vi "Main-GUI.vi"() -> ()   [LabVIEW 2021]
uses:
  Controls/Command_cluster.ctl
  Controls/Command_Enum.ctl
  Controls/AR-msg-variables.ctl
  Controls/AR-com-ports.ctl
  Controls/AR-instrument-refs.ctl
  C:/Projects/Automation/nLight Laser/nlight_dll/altaAPI.dll
  Automation/nLight Laser/nlight_dll/altaAPI.dll
  Controls/AR-axis-parameters.ctl
  Automation/Zaber Stage/Controls/Zaber-parameters.ctl
  Controls/AR-Interlock-Data.ctl
  Automation/nLight Laser/Controls/CW-Laser-params.ctl
  Automation/nLight Laser/Controls/Status-flags.ctl
  Automation/nLight Laser/Controls/nLight-beam-modes.ctl
  Controls/AR-Interlock-monitor-comands.ctl
  Automation/nLight Laser/Controls/nLight-wait-states.ctl
  <instrlib>/Zaber A Series/Zaber A Series.lvlib
panel:
  out "Accel Activ":bool
  out "msg-var at exit":T1={"Run Rcp"=FALSE, "Rcp Stopped"=FALSE, "Err Device"="", "Run Axis Loop"=TRUE}
  in  "Simulate Laser":bool
  out "error out":errorcluster
  in  "Axis params":T2={"X"={"Device (dev axis)"="1 3", "Lockstep Group (1)"=1, "Units"=enum."millimeters", "Microstep Size"=4.21875, "Move (units)"=1500.0, "Direction(-1,1)"=1, "Speed (units/s)"=0.0}, "Y"={"Device (dev axis)"="1", "Lockstep Group (1)"=1, "Units"=enum."millimeters", "Microstep Size"=0.496094, "Move (units)"=0.0, "Direction(-1,1)"=1, "Speed (units/s)"=0.0}}
  in  "Tab Control":T4(tab)=enum."SETTINGS (AXIS / SCRIPT)"
  in  "Start Y Position":dbl=85.0
  in  "Re-test gating":bool
  in  "X Axis Initial Test Parameters":T3={"Device (dev axis)"="1 3", "Lockstep Group (1)"=1, "Units"=enum."millimeters", "Microstep Size"=4.21875, "Move (units)"=1500.0, "Direction(-1,1)"=1, "Speed (units/s)"=0.0}
  out "MCU INLK":bool=TRUE
  in  "Init":bool=TRUE
  out "Laser OK":bool
  in  "Com ports":T5={"Zaber Com"="COM3", "MCU Com"="COM5", "Laser IP"="172.30.0.50", "Laser Com"=""}
  in  "Recipe (csv)":path=path "C:/Projects/Alpha Redux/test-scrypt-1.csv"
  out "Zaber OK":bool=TRUE
  out "Controll Interface":i32(ring) items=["HW", "API", "CLI", "INET, CONTROL_INT_MASK"]
  out "External Gate":bool
  out "Profile Mode":bool
  out "Gating Timedout":bool
  out "X Position Triggered":dbl
  out "Delta Time (mS)":dbl
  out "MCU Gating Flags":T6
  in  "Save script":bool
  in  "Load script":bool
  in  "Script":T7[](array[typedef])=[{"Step#"=10.0, "Commands"=enum."Home All", "Parameter1"=0.0, "Parameter2"=0.0, "Parameter3"=0.0}, {"Step#"=20.0, "Commands"=enum."Y Move Rel", "Parameter1"=20.0, "Parameter2"=1.0, "Parameter3"=0.0}, {"Step#"=30.0, "Commands"=enum."Wait", "Parameter1"=500.0, "Parameter2"=0.0, "Parameter3"=0.0}, {"Step#"=40.0, "Commands"=enum."X Move Abs", "Parameter1"=300.0, "Parameter2"=0.0, "Parameter3"=0.0}, {"Step#"=50.0, "Commands"=enum."Wait", "Parameter1"=1000.0, "Parameter2"=0.0, "Parameter3"=0.0}, {"Step#"=60.0, "Commands"=enum."Y Move Rel", "Parameter1"=10.0, "Parameter2"=-1.0, "Parameter3"=0.0}, {"Step#"=70.0, "Commands"=enum."Wait", "Parameter1"=500.0, "Parameter2"=0.0, "Parameter3"=0.0}, {"Step#"=80.0, "Commands"=enum."X Move Abs", "Parameter1"=50.0, "Parameter2"=0.0, "Parameter3"=0.0}, {"Step#"=90.0, "Commands"=enum."Wait", "Parameter1"=1000.0, "Parameter2"=0.0, "Parameter3"=0.0}, {"Step#"=100.0, "Commands"=enum."Repeat", "Parameter1"=20.0, "Parameter2"=5.0, "Parameter3"=0.0}, {"Step#"=110.0, "Commands"=enum."Y Move Abs", "Parameter1"=10.0, "Parameter2"=0.0, "Parameter3"=0.0}, {"Step#"=120.0, "Commands"=enum."End", "Parameter1"=0.0, "Parameter2"=0.0, "Parameter3"=0.0}]
  in  "Y Microstep Size":dbl=0.496094
  in  "X Microstep Size":dbl=4.21875
  in  "Y (dev axis)":string="1"
  in  "X (dev axis)":string="1 3"
  in  "Select Units":T9(ring)=enum."millimeters"
  in  "Zaber settings":bool
  out "Device Info":T10(array[cluster])=[{"Motion Type"="Linear", "Device Name"="X-MCC3 (rev 2) Controller + LRQ150BL-DE51T10A", "Microstep Size"=0.49609375000198436}, {"Motion Type"="Linear", "Device Name"="X-MCC3 (rev 2) Controller + LRQ150BL-DE51T10A", "Microstep Size"=0.49609375000198436}, {"Motion Type"="Linear", "Device Name"="X-MCC3 (rev 2) Controller + BLQ2095-E01T3A", "Microstep Size"=4.2187499996625}] {"Microstep Size" format="%#_6f"}
  out "Devices":string[](array[string])=["1"]
  out "Axis":string[](array[string])=["3"]
  out "Mode RDY":bool
  in  "Beam-profile(0-6)":T11
  in  "Speed mm/s":dbl=500.0
  in  "Clear":bool
  in  "Request":bool
  out "Gating Data":T12={"Application"="", "Msg#"=0, "uS time"=0, "Gate"=TRUE, "Head"=TRUE, "Head Old"=FALSE, "Chamber Ena"=FALSE, "Profiler Ena"=FALSE, "OPower Ena"=FALSE, "Gate Ena"=FALSE, "Time Delta (mS)"=0.0, "Head F Edge"=FALSE} {"Time Delta (mS)" format="%#_3f"}
  out "MCU Gating Raw Output":string
  out "Laser Msg Log":string
  in  "Laser Params":T13={"Power(W)"=30.0, "Duty(%)"=5.0, "Freq(Hz)"=1000.0}
  in  "SysON":bool
  in  "ENA":bool
  in  "Set Laser Params":bool caption="Set"
  out "Laser Status":T14
  out "Current Y Pos":dbl
  in  "Y Home":bool
  in  "Y Abs":bool
  in  "Y Abs Units":dbl=50.0
  out "Current X Pos":dbl=-3.9234375
  in  "Stop":bool
  in  "X Home":bool
  in  "X Abs":bool
  in  "X Abs Units":dbl=500.0
  in  "Y Units":dbl=1.0
  in  "X Units":dbl=10.0
  in  "Y Fw":bool
  in  "Y Back":bool
  in  "X Fw":bool
  in  "X Back":bool
  in  "EMIT!":bool
  in  "Head Flag\nLenght (mm)":dbl=100.0
  in  "Run script":bool
  in  "Stop":bool
  in  "Next":bool
  in  "Step":bool
  out "Y Position":dbl
  out "X Position":dbl
  out "Gate Trigger":cluster{dbl[], i16[]}(graph) caption="XY Graph - Light"
  out "Speeds (m/s)":dbl[](array[numeric])
  out "X Axis Pos/Speed":cluster{u32[], dbl[]}(graph) caption="XY Graph - Light"
  in  "Select":bool
  out "Laser Status":T14
  out "Laser Power (W)":dbl
  out "Laser Duty (%)":dbl
  out "Next command":T7
  in  "Target Time (s)":dbl=1.0
  in  "Accel COM":refnum<visa-resource-name>
  in  "Accel CSV File":path=path "C:/Users/cleanroom/Desktop/Accelerometer Files/Test1.csv"
  in  "Accel Ena":bool caption="ENABLE"
  out "File OK":bool
  out "Com\nError":bool
  out "Instr Refs":T15={"Zaber Com"="COM21", "MCU Com"="COM22", "LaserSysRef Out"=refnum, "LaserControl Ref Out"=refnum}
  in  "error in":errorcluster
  out "msg-var":T1={"Run Rcp"=FALSE, "Rcp Stopped"=FALSE, "Err Device"="", "Run Axis Loop"=TRUE}
  in  "Quit":bool
  out "Action":string="Quit"
  # "Emit not used\nwith EXT TRIG"
  # "EMIT! will work\nonly in GUI/CLI mode without EX GATE"
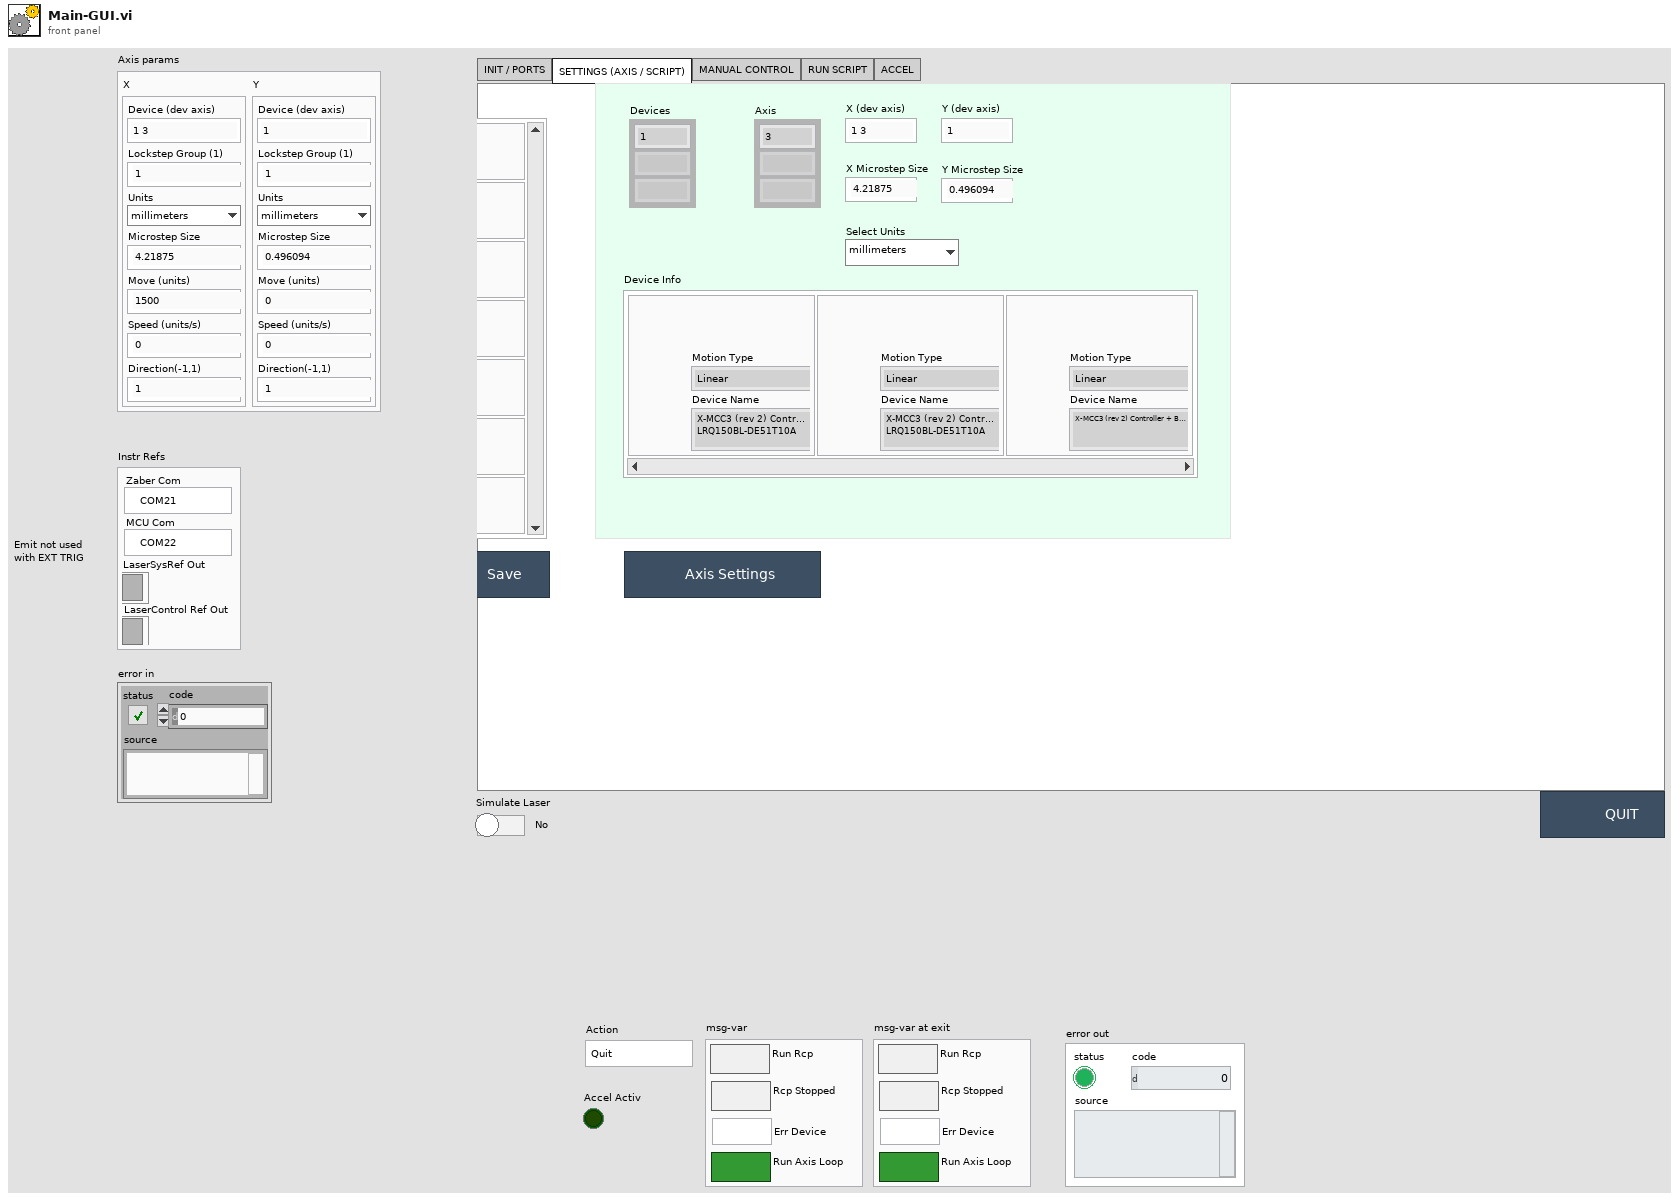
[diagram p1: front panel]
types:
  T1 = typedef "AR-msg-variables.ctl" = cluster{"Run Rcp":bool, "Rcp Stopped":bool, "Err Device":string, "Run Axis Loop":bool}
  T2 = typedef "AR-axis-parameters.ctl" = cluster{"X":T3, "Y":T3}
  T3 = typedef "Zaber-parameters.ctl" = cluster{"Device (dev axis)":string, "Lockstep Group (1)":u8, "Units":enum16{"microsteps", "microns", "millimeters", "inches", "degrees"}, "Microstep Size":dbl, "Move (units)":dbl, "Direction(-1,1)":i32, "Speed (units/s)":dbl}
  T4 = enum32{"INIT / PORTS", "SETTINGS (AXIS / SCRIPT)", "MANUAL CONTROL", "RUN SCRIPT", "ACCEL"}
  T5 = typedef "AR-com-ports.ctl" = cluster{"Zaber Com":refnum<visa-resource-name>, "MCU Com":refnum<visa-resource-name>, "Laser IP":string, "Laser Com":refnum<visa-resource-name>}
  T6 = cluster{"Chamber Ena":bool, "Profiler Ena":bool, "OPower Ena":bool}
  T7 = typedef "Command_cluster.ctl" = cluster{"Step#":dbl, "Commands":T8, "Parameter1":dbl, "Parameter2":dbl, "Parameter3":dbl}
  T8 = typedef "Command_Enum.ctl" = enum16{"End", "Home All", "X Home", "Y Home", "X Move Rel", "X Move Abs", "Y Move Rel", "Y Move Abs", "Wait", "Repeat", "Reset Intlk Timer", "Laser Sys ON", "Laser ENA"}
  T9 = enum16{"microsteps", "microns", "millimeters", "inches", "degrees"}
  T10 = cluster{"Motion Type":string, "Device Name":string, "Microstep Size":dbl}[]
  T11 = typedef "nLight-beam-modes.ctl" = enum32{"0/100 single-mode", "30/70", "40/60", "50/50", "60/40", "80/20", "90/10 max donut"}
  T12 = typedef "AR-Interlock-Data.ctl" = cluster{"Application":string, "Msg#":i32, "uS time":u32, "Gate":bool, "Head":bool, "Head Old":bool, "Chamber Ena":bool, "Profiler Ena":bool, "OPower Ena":bool, "Gate Ena":bool, "Time Delta (mS)":dbl, "Head F Edge":bool}
  T13 = typedef "CW-Laser-params.ctl" = cluster{"Power(W)":dbl, "Duty(%)":dbl, "Freq(Hz)":dbl}
  T14 = typedef "Status-flags.ctl" = cluster{"SystemOn":bool, "Enabled":bool, "LaserOn":bool, "Standby":bool, "Interlock":bool, "Error":bool, "Warning":bool, "Fault":bool}
  T15 = typedef "AR-instrument-refs.ctl" = cluster{"Zaber Com":refnum<visa-resource-name>, "MCU Com":refnum<visa-resource-name>, "LaserSysRef Out":refnum<k24>, "LaserControl Ref Out":refnum<k24>}
  T16 = enum32{"INIT / PORTS", "SETTINGS (AXIS / SCRIPT)", "MANUAL CONTROL", "RUN SCRIPT"}
  T17 = enum32{"Page Enabled", "Page Disabled", "Page Disabled & Grayed"}
  T18 = typedef "AR-Interlock-monitor-comands.ctl" = enum16{"Init", "Request", "Poll Serial", "Close", "Clear Data"}
  T19 = enum8{"Enabled", "Disabled", "Disabled and Grayed Out"}
  T20 = typedef "nLight-wait-states.ctl" = enum16{"Wait SysON", "Wait ENA", "Wait SysOFF", "Wait DIS", "No Wait"}
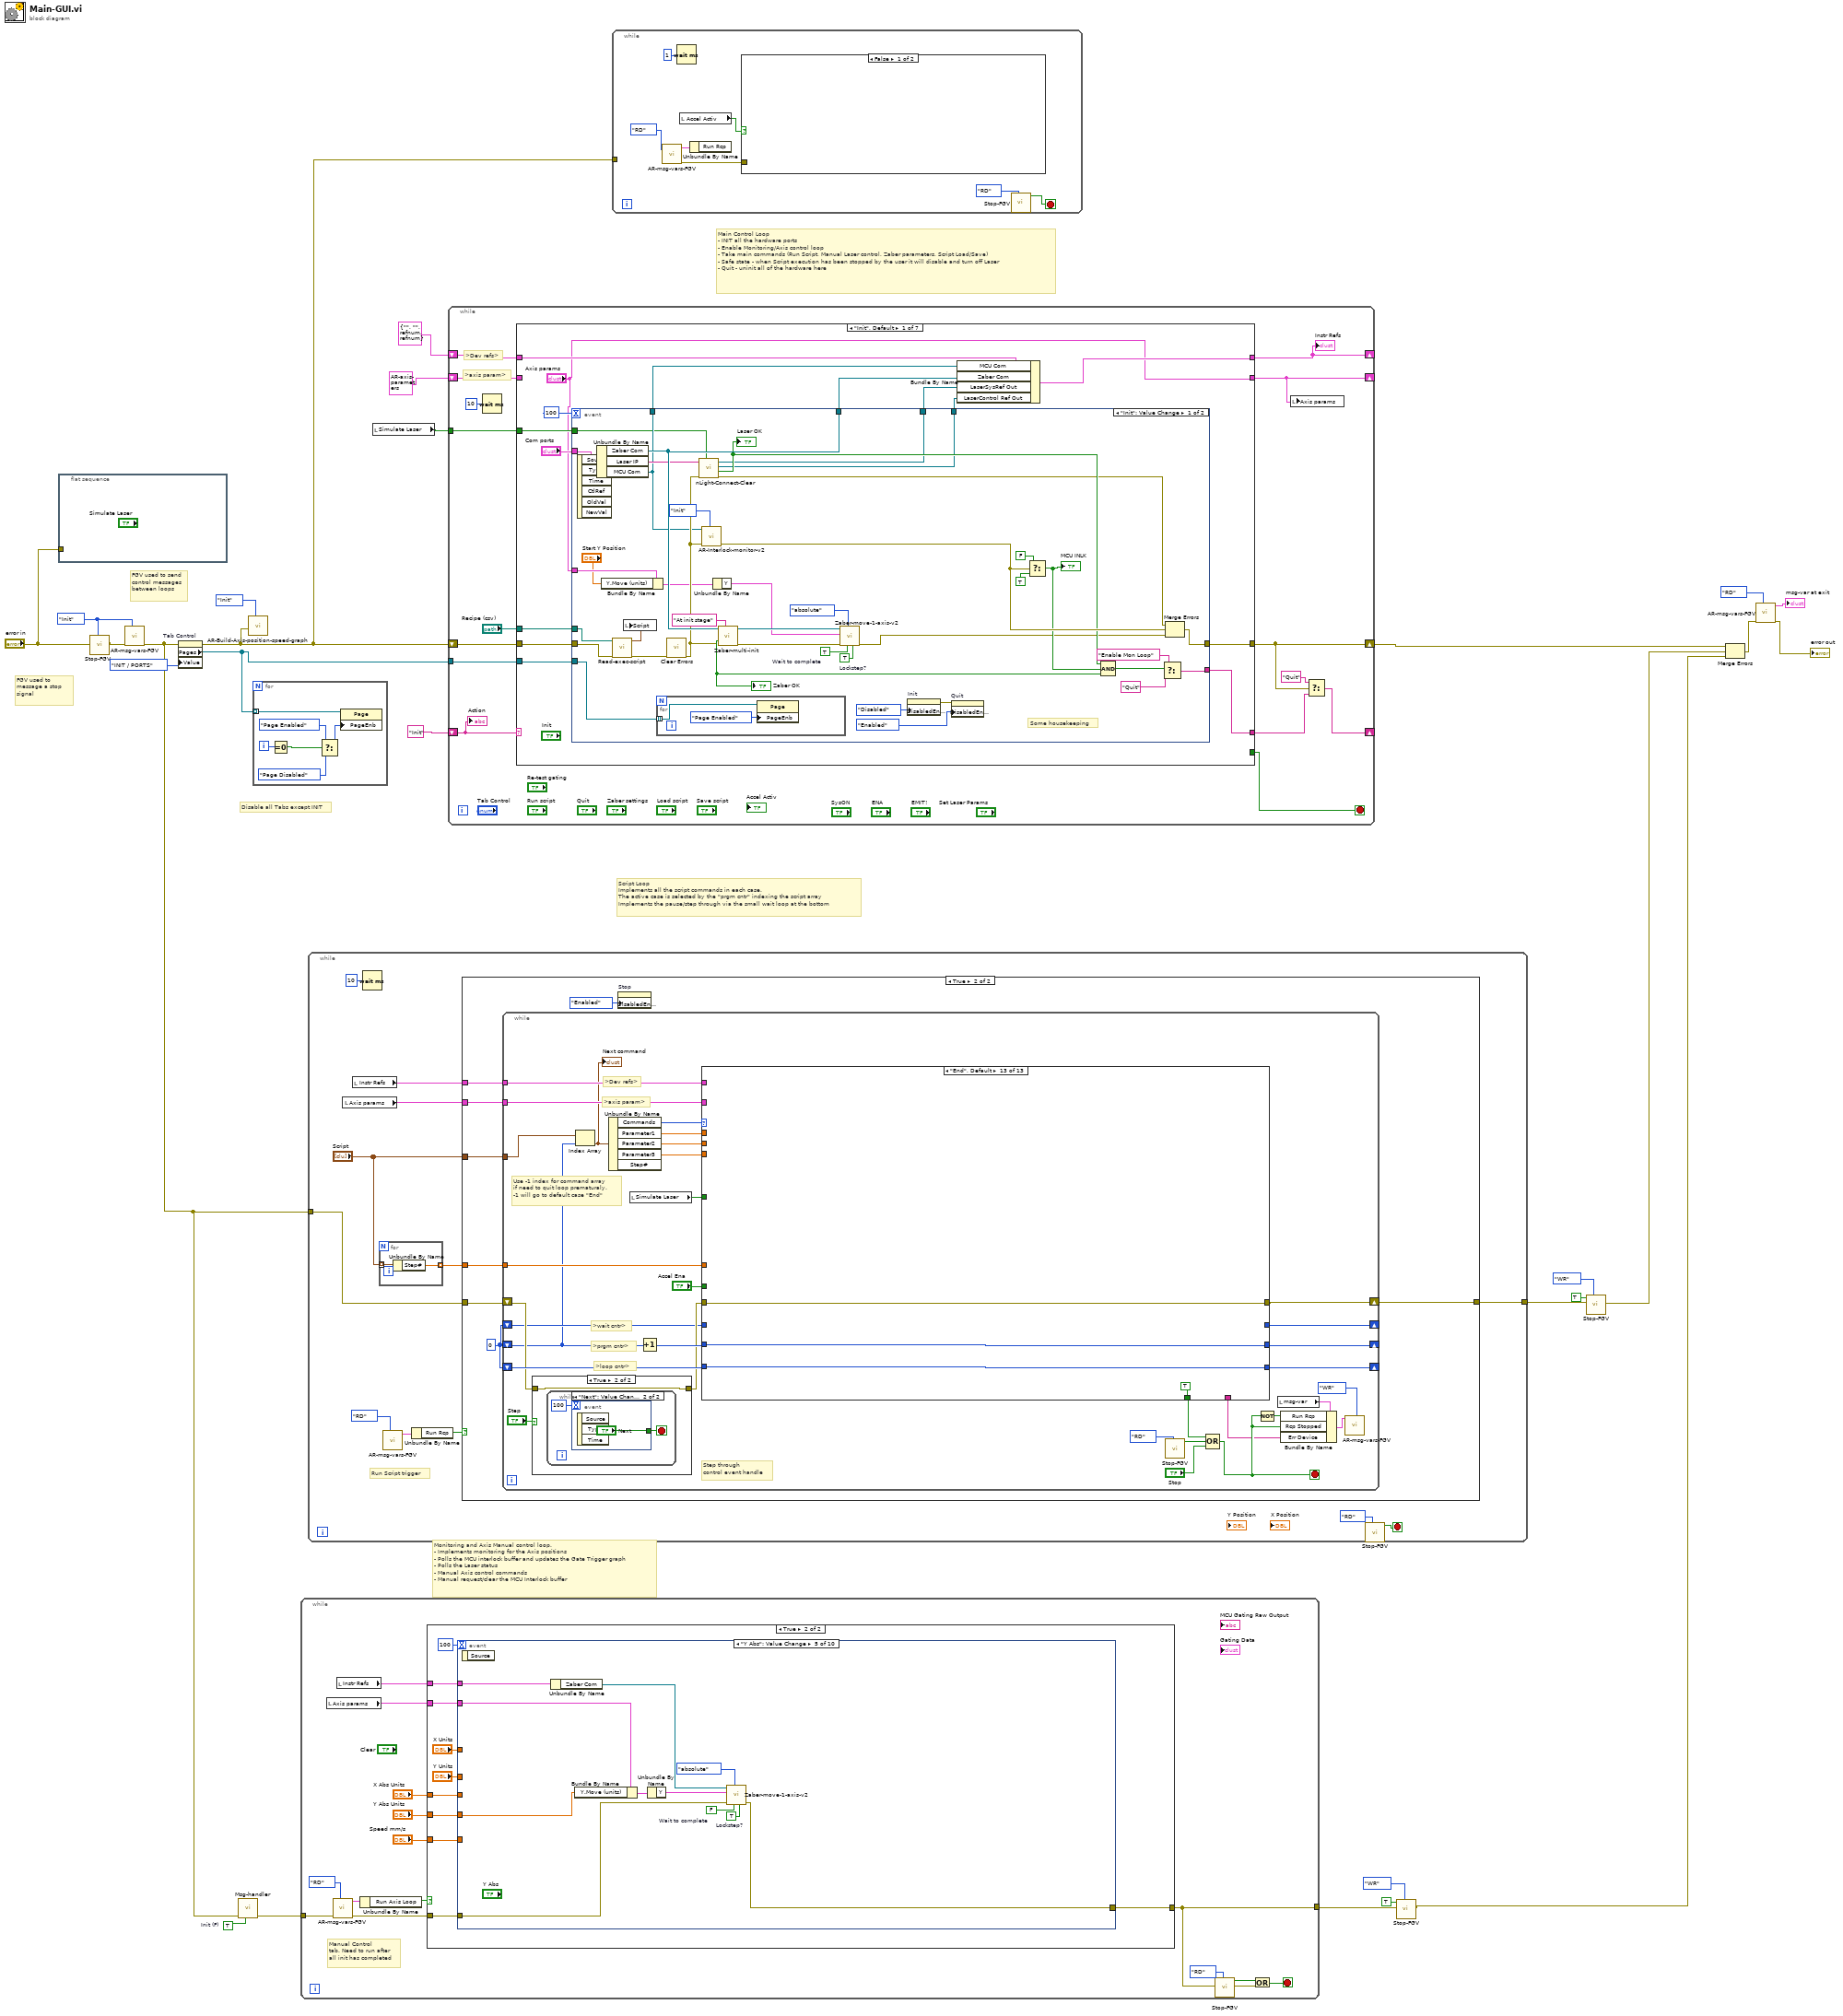
[diagram p0: block diagram]
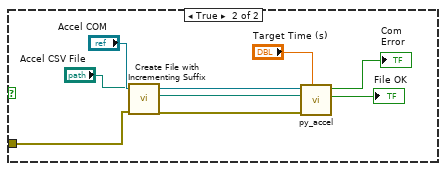
[diagram p2: hidden frame]
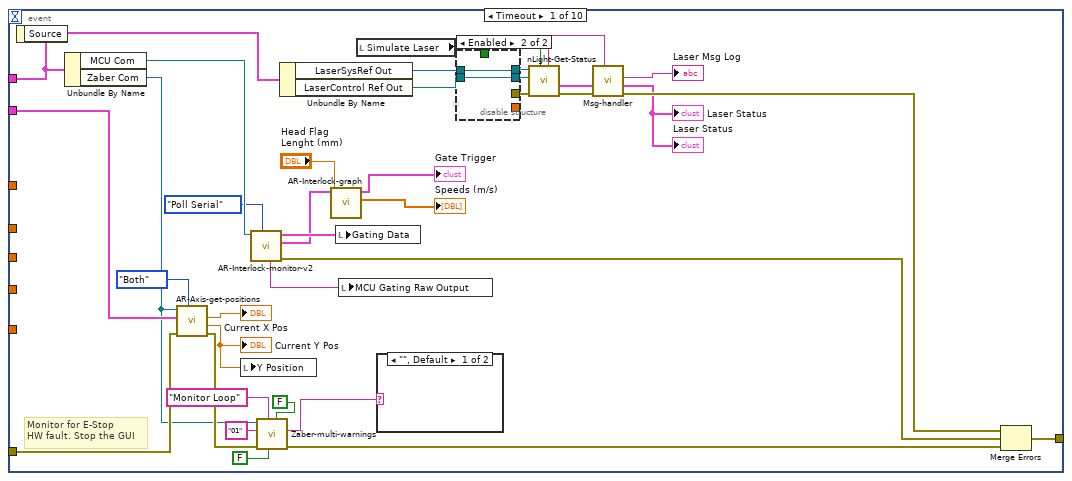
[diagram p4: hidden frame]
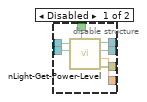
[diagram p5: hidden frame]
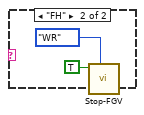
[diagram p6: hidden frame]
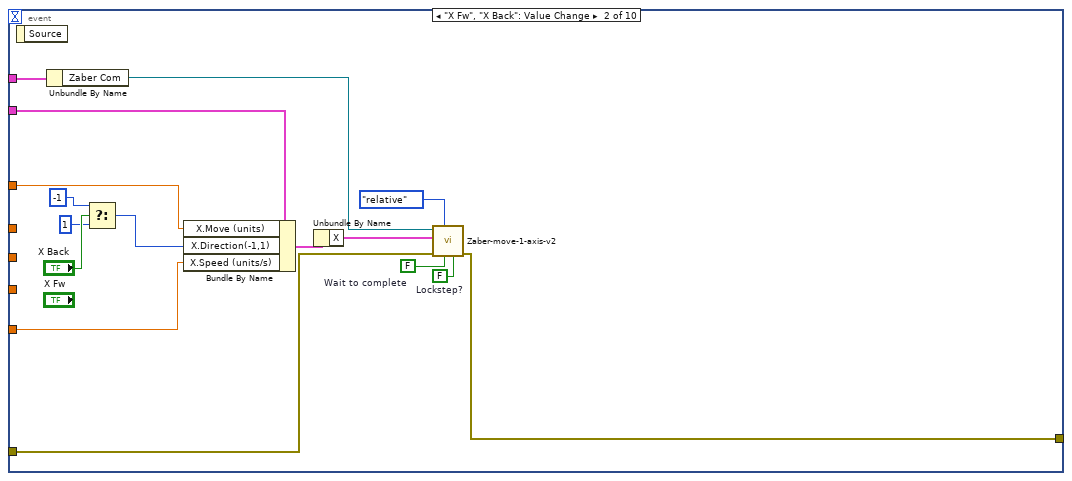
[diagram p7: hidden frame]
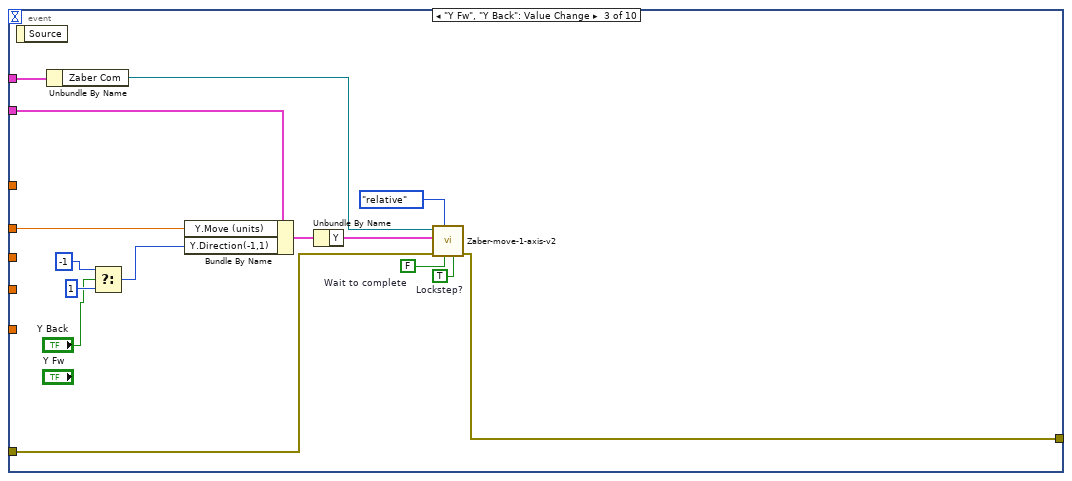
[diagram p8: hidden frame]
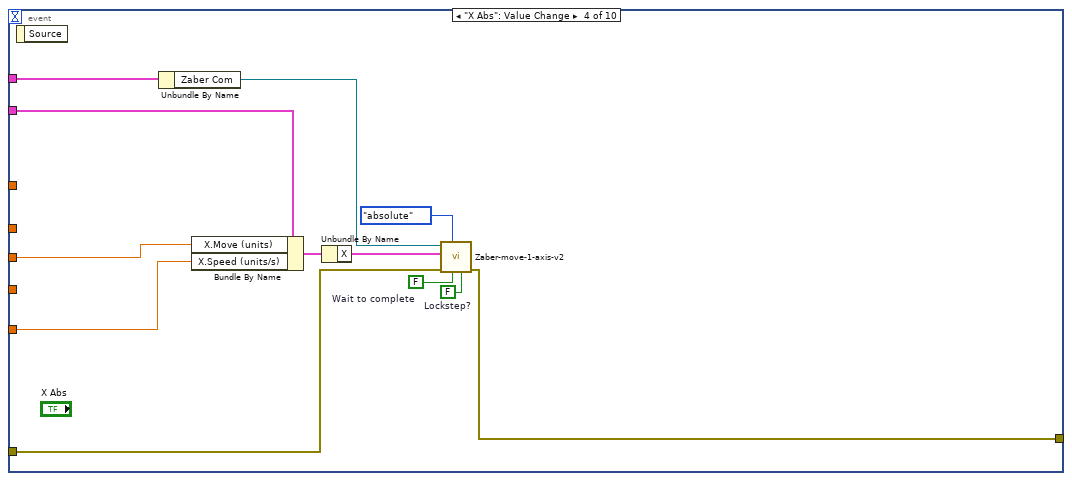
[diagram p9: hidden frame]
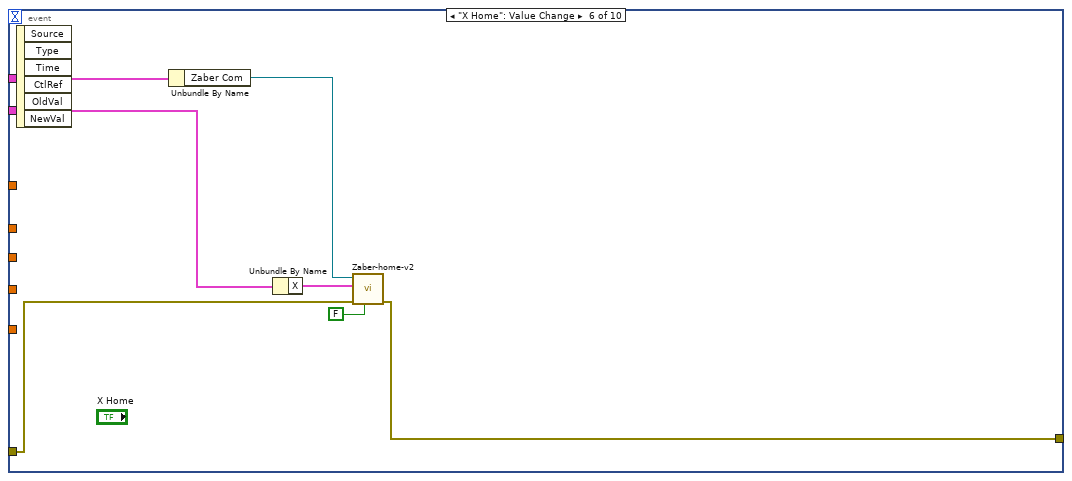
[diagram p10: hidden frame]
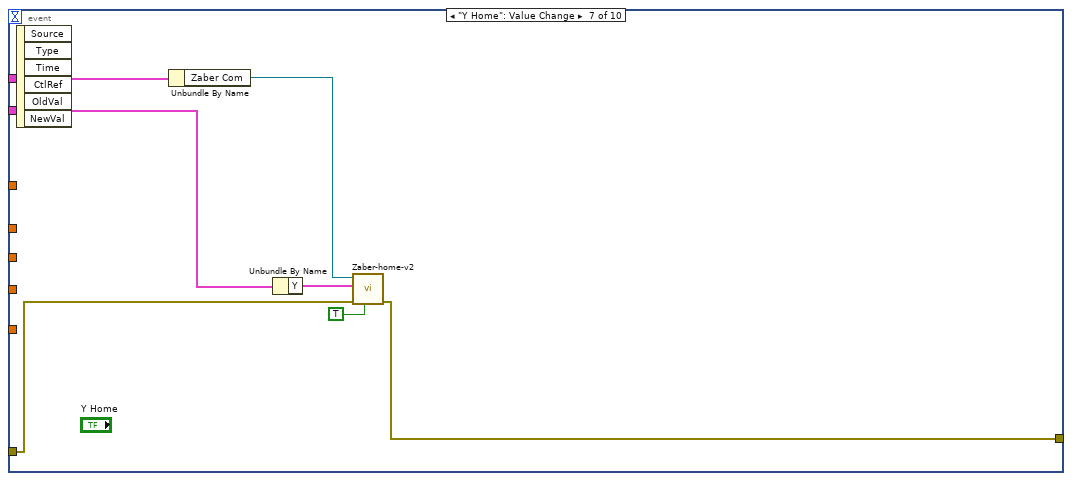
[diagram p11: hidden frame]
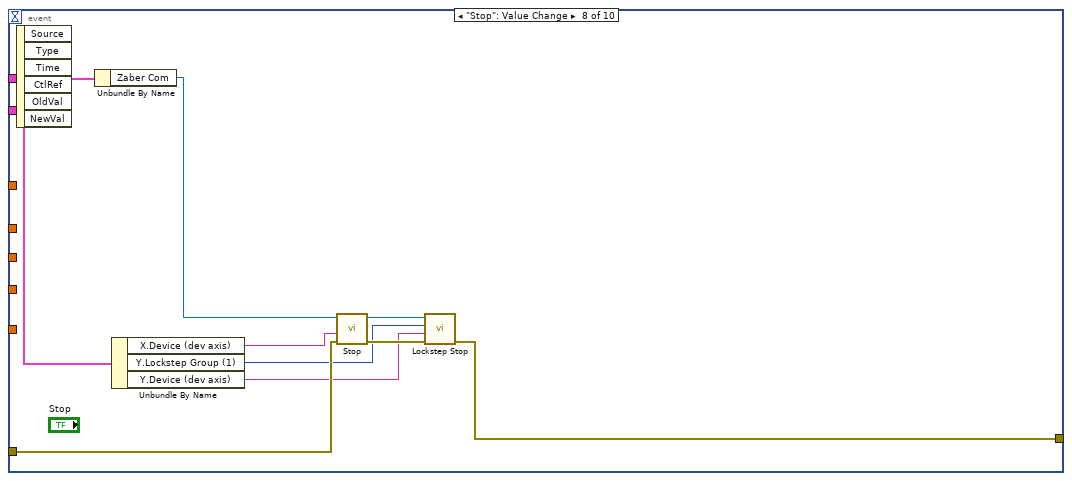
[diagram p12: hidden frame]
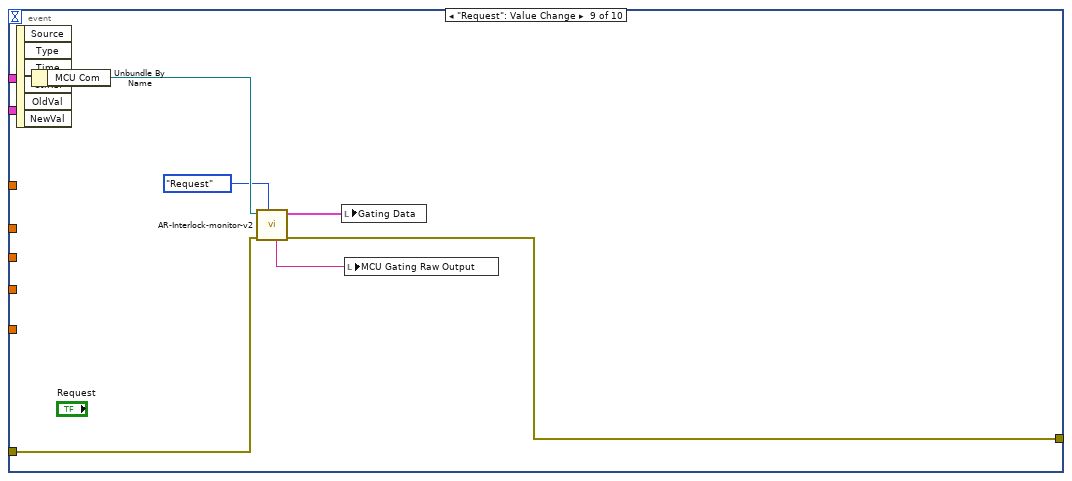
[diagram p13: hidden frame]
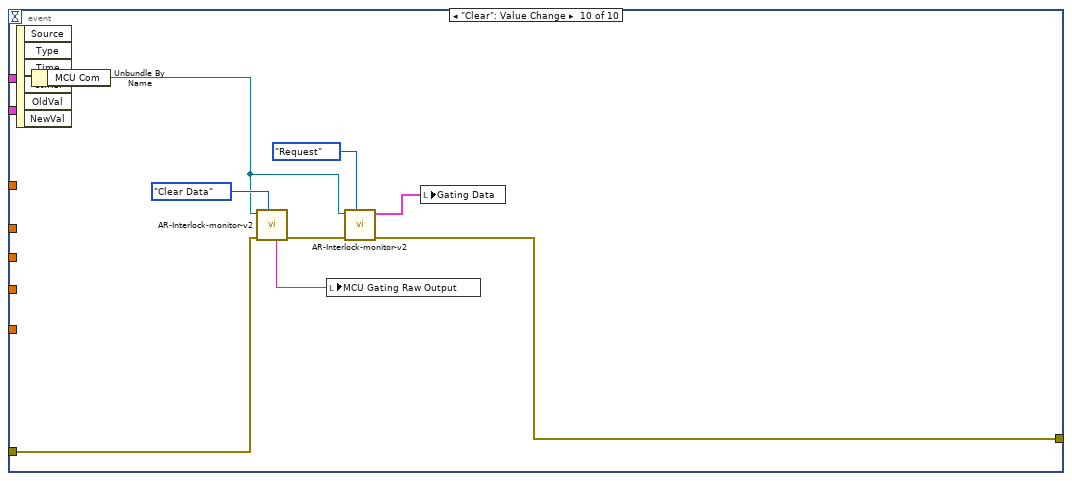
[diagram p14: hidden frame]
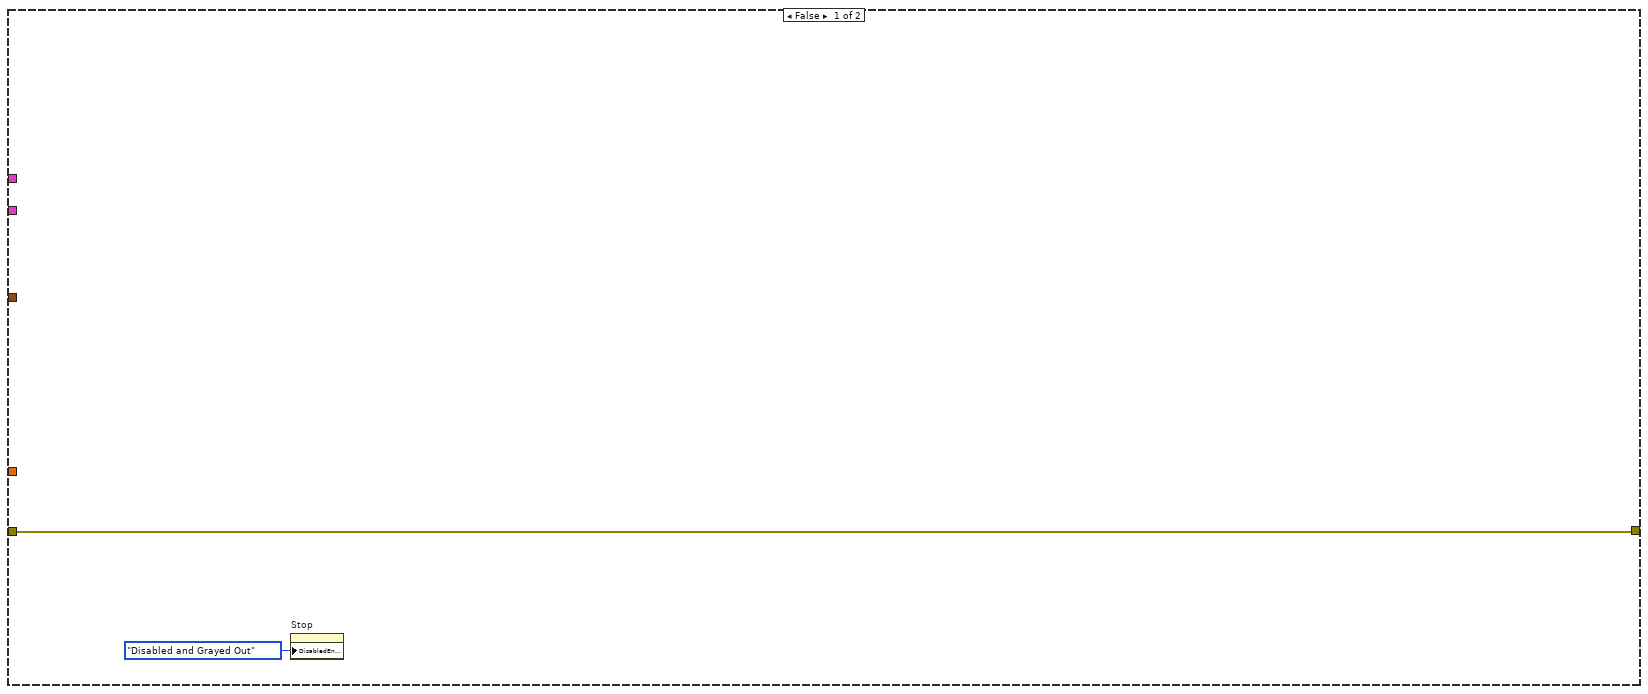
[diagram p15: hidden frame]
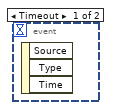
[diagram p17: hidden frame]
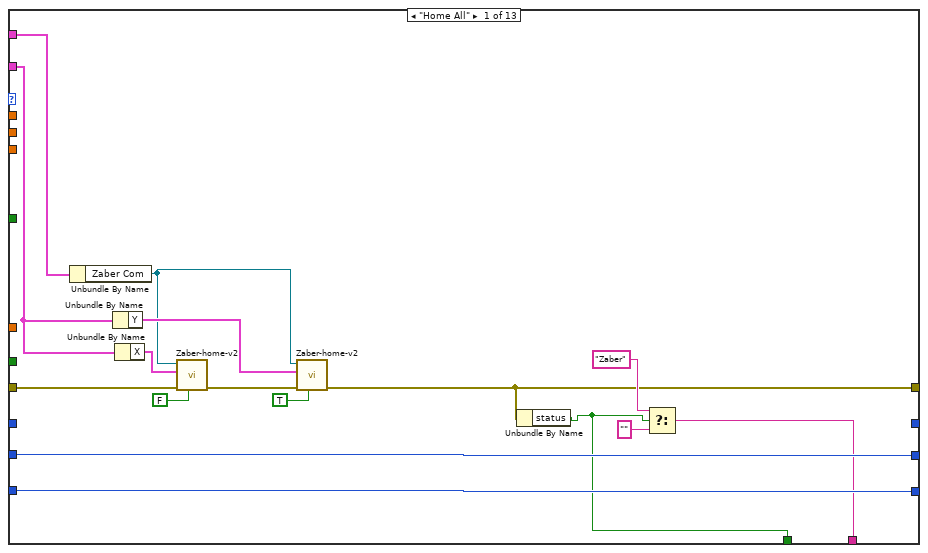
[diagram p18: hidden frame]
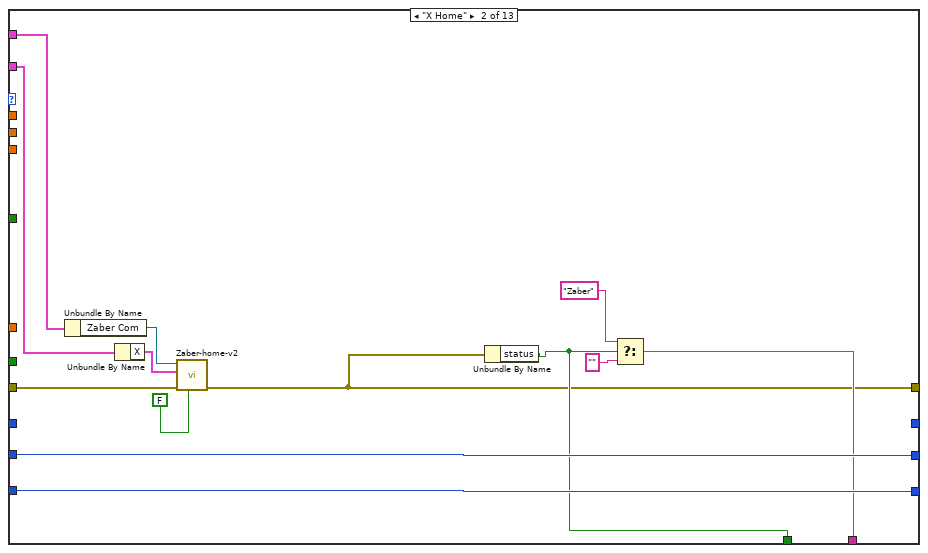
[diagram p19: hidden frame]
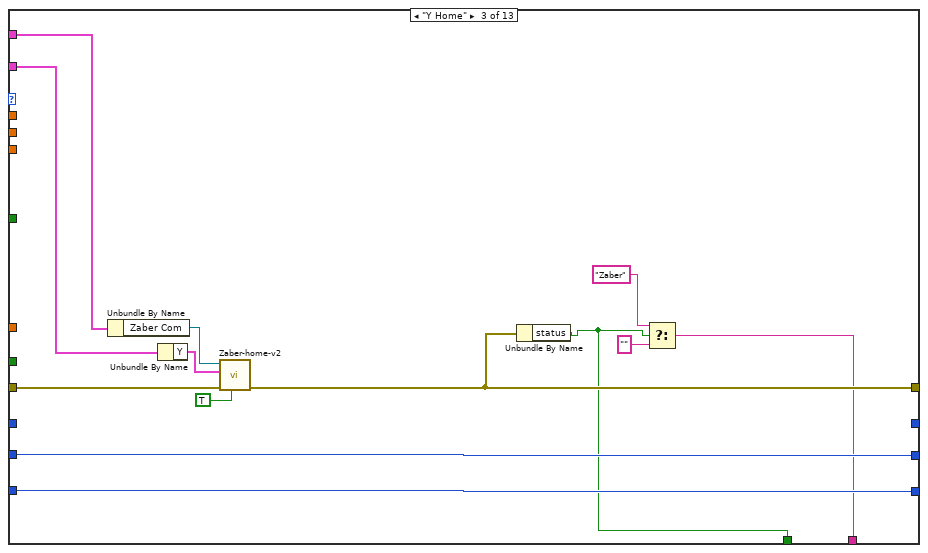
[diagram p20: hidden frame]
diagram:
  w19 = TRUE  # Init (F)
  w25 = enum16{"Init", "WR", "RD"}."Init" ("Action (RD)")
  # "Monitoring and Axis Manual control loop.\n- Implements monitoring for the Axis positions\n- Polls the MCU interlock buffer and updates the Gate Trigger graph\n- Polls the Laser status\n- Manual Axis control commands\n- Manual request/clear the MCU Interlock buffer"
  # "Main Control Loop\n- INIT all the hardware ports \n- Enable Monitoring/Axis control loop\n- Take main commands (Run Script, Manual Laser control, Zaber parameters, Script Load/Save)\n- Safe state - when Script execution has been stopped by the user it will disable and turn off Laser\n- Quit - uninit all of the hardware here"
  # "Disable all Tabs except INIT"
  # "FGV used to send control messages between loops"
  # "FGV used to \nmessage a stop\nsignal"
  # "Script Loop\nImplements all the script commands in each case.\nThe active case is selected by the \"prgm cntr\" indexing the script array\nImplements the pause/step through via the small wait loop at the bottom"
  n1 = flat-sequence {
    tunnel: "error in" -> [_]
    frame #0 {
    }
  }
  n2 = call "Stop-FGV.vi"("Action (RD)"=w25, "error in"="error in") -> ("error out"=w26:errorcluster)  [unwired: 8 in, 1 out]
  n3 = call "AR-msg-vars-FGV.vi"("Action"=w25, "error in"=w26) -> ("error out"=w18:errorcluster)  [unwired: 8 in, 1 out]
  n4 = property on="Tab Control" class="TabCtl (strict)"(error in=w18, "Value"=T16."INIT / PORTS" ("Tab Control")) -> (error out=w1:errorcluster, "Pages"=w22:refnum<vi>[])  [unwired: 1 in, 1 out]
  n5 = call "Msg-handler.vi"("Init (F)"=w19, "error in"=w18) -> ("error out"=w17:errorcluster)  [unwired: 6 in, 3 out]
  n6 = call "AR-Build-Axis-position-speed-graph.vi"("Action"=enum16{"Init", "WR", "RD"}."Init", "error in (no error)"=w1) -> ()  [unwired: 9 in, 1 out]
  n7 = for {
    tunnel: w22 -> [w33] mode=indexing
    i -> [w32]
    n8 = Equal To 0?(x=w32) -> (x = 0?=w31:bool)
    n9 = Select(t=T17."Page Enabled" ("Page Enabled State"), s=w31, f=T17."Page Disabled" ("Page Enabled State")) -> (s? t:f=w28:T17)
    n10 = property class="Page"(reference=w33, "PageEnb"=w28) -> ()  [unwired: 1 in, 2 out]
  }
  n11 = while {
    tunnel: w17 -> [w42]
    tunnel: [w36] -> w11
    stop <- w40 stop-if-true
    # "Manual Control\ntab. Need to run after\nall init has completed"
    n12 = local read "Axis params"() -> (w43:T2)
    n13 = call "AR-msg-vars-FGV.vi"("Action"=enum16{"Init", "WR", "RD"}."RD", "error in"=w42) -> ("error out"=w41:errorcluster, "msg-var"=w47:T1)  [unwired: 8 in]
    n14 = local read "Instr Refs"() -> (w44:T15)
    n15 = Unbundle By Name(w47) -> ("Run Axis Loop"=w45:bool)
    n16 = case shown="True" w45 {
      tunnel: w44 -> [_ w59]
      tunnel: w43 -> [_ w58]
      tunnel: w41 -> [w49 w57]
      tunnel: [w49 w56] -> w36
      tunnel: "X Abs Units" -> [_ w52]
      tunnel: "Y Abs Units" -> [_ w51]
      tunnel: "Speed mm/s" -> [_ w50]
      frame False {
      }
      frame True {
        # "Run Sequence"
        n17 = event shown="[4] \"Y Abs\": Value Change" {
          selector: _ -> [_ _ _ _ _ _ _ _ _ _]
          dyn-events: _ -> [_ _ _ _ _ _ _ _ _ _]
          timeout: 100 -> [_ _ _ _ _ _ _ _ _ _]
          tunnel: w59 -> [w78 w112 w128 w143 w154 w164 w171 w184 w187 w199]
          tunnel: w58 -> [w94 w113 w129 w144 w155 w163 w170 w178 _ _]
          tunnel: w57 -> [w93 w110 w126 w140 w152 w162 w169 w181 w189 w200]
          tunnel: [w88 w109 w125 w139 w151 w161 w168 w179 w188 w196] -> w56
          tunnel: "Y Units" -> [_ _ w123 _ _ _ _ _ _ _]
          tunnel: "X Units" -> [_ w108 _ _ _ _ _ _ _ _]
          tunnel: w52 -> [_ _ _ w141 _ _ _ _ _ _]
          tunnel: w51 -> [_ _ _ _ w150 _ _ _ _ _]
          tunnel: w50 -> [_ w107 _ w138 _ _ _ _ _ _]
          event Timeout {
            # "Monitor for E-Stop\nHW fault. Stop the GUI"
            n18 = event-data() -> ()  [unwired: 1 in, 1 out]
            n19 = Unbundle By Name(w78) -> ("MCU Com"=w91:refnum<visa-resource-name>, "Zaber Com"=w66:refnum<visa-resource-name>)
            n20 = call "AR-Axis-get-positions.vi"("Select"=enum16{"X Axis", "Y Axis", "Both"}."Both", "error in"=w93, "Axis params"=w94, "Port In"=w66) -> ("error out"=w67:errorcluster, "Y Pos"=w82:dbl, "X Pos"=→"Current X Pos":dbl)  [unwired: 4 in, 1 out]
            "Current Y Pos" <- w82
            n21 = local write "Y Position"(w82) -> ()
            n22 = call "AR-Interlock-monitor-v2.vi"("Action"=AR-Interlock-monitor-comands."Poll Serial", "Inlk Com"=w91) -> ("error out"=w89:errorcluster, "Intlk Data Array"=w85:T12[], "Intlk Data"=w86:T12, "Raw Output"=w87:string)  [unwired: 5 in, 1 out]
            n23 = call "Zaber-multi-warnings.vi"("Log?"=FALSE, "Msg?"=FALSE, "LogSource"="Monitor Loop", "error in"=w67, "Device"="01", "Com Port"=w66) -> ("error out"=w62:errorcluster, "Warning Flag"=w61:string)  [unwired: 2 in, 2 out]
            n24 = Unbundle By Name(w78) -> ("LaserSysRef Out"=w74:refnum<k24>, "LaserControl Ref Out"=w72:refnum<k24>)
            n25 = call "AR-Interlock-graph.vi"("Flag Lenght (mm)"="Head Flag\nLenght (mm)", "Intlk Data Array"=w85) -> ("Speeds (m/s)"=→"Speeds (m/s)":dbl[], "Gate"=→"Gate Trigger":cluster{dbl[], i16[]})  [unwired: 7 in, 1 out]
            n26 = local write "Gating Data"(w86) -> ()
            n27 = local write "MCU Gating Raw Output"(w87) -> ()
            n28 = local read "Simulate Laser"() -> (w69:bool)
            n29 = case shown="\"\", Default" w61 {
              frame "", Default {
              }
              frame "FH" {
                n30 = call "Stop-FGV.vi"("Action (RD)"=enum16{"Init", "WR", "RD"}."WR", "Action"=TRUE) -> ()  [unwired: 8 in, 2 out]
              }
            }
            n31 = disable-structure shown="Enabled" {
              disable-tunnel: w74 -> [w102 w103]
              disable-tunnel: [w101 w103] -> w73
              disable-tunnel: w72 -> [w100 w104]
              disable-tunnel: [w99 w104] -> w71
              disable-tunnel: [w98 _] -> w70
              disable-tunnel: [w97 _] -> _
              disable-tunnel: w69 -> [w96 _]
              frame Disabled {
                n32 = call "nLight-Get-Power-Level.vi"("Simulate (F)"=w96, "LaserControl Ref"=w100, "LaserSysRef"=w102) -> ("error out"=w98:errorcluster, "PowerOutput"=w97:dbl, "LaserControl Ref Out"=w99:refnum<k24>, "LaserSysRef Out"=w101:refnum<k24>)  [unwired: 5 in]
              }
              frame Enabled {
              }
            }
            n33 = call "nLight-Get-Status.vi"("Simulate (F)"=w69, "error in"=w70, "LaserControl Ref"=w71, "LaserSysRef"=w73) -> ("error out"=w79:errorcluster, "Status-flags"=w80:T14, "Msg"=w81:string)  [unwired: 2 in, 3 out]
            n34 = call "Msg-handler.vi"("Msg"=w81, "error in"=w79, "Status-flags"=w80) -> ("error out"=w76:errorcluster, "Status-flags Out"=→"Laser Status" →"Laser Status":T14, "Msg log"=→"Laser Msg Log":string)  [unwired: 5 in, 1 out]
            n35 = Merge Errors(w76, w89, w62) -> (w88:errorcluster)
          }
          event "X Fw", "X Back": Value Change {
            w117 = FALSE  # Wait to complete
            w118 = FALSE  # Lockstep?
            n36 = event-data() -> ()  [unwired: 1 in, 1 out]
            n37 = Unbundle By Name(w112) -> ("Zaber Com"=w111:refnum<visa-resource-name>)
            n38 = Select(t=-1 ("Direction(-1,1)"), s="X Back", f=1) -> (s? t:f=w121:i32)
            n39 = Bundle By Name(cluster=w113, "X.Move (units)"=w108, "X.Direction(-1,1)"=w121, "X.Speed (units/s)"=w107) -> (w114:T2)
            n40 = Unbundle By Name(w114) -> ("X"=w115:T3)
            n41 = call "Zaber-move-1-axis-v2.vi"("Lockstep?"=w118, "Wait to complete"=w117, "Movement Type"=enum16{"relative", "absolute"}."relative", "error in"=w110, "Zaber parameters"=w115, "Port In"=w111) -> ("error out"=w109:errorcluster)  [unwired: 3 in, 2 out]
          }
          event "Y Fw", "Y Back": Value Change {
            w133 = FALSE  # Wait to complete
            w134 = TRUE  # Lockstep?
            n42 = event-data() -> ()  [unwired: 1 in, 1 out]
            n43 = Unbundle By Name(w128) -> ("Zaber Com"=w127:refnum<visa-resource-name>)
            n44 = Select(t=-1 ("Direction(-1,1)"), s="Y Back", f=1) -> (s? t:f=w137:i32)
            n45 = Bundle By Name(cluster=w129, "Y.Move (units)"=w123, "Y.Direction(-1,1)"=w137) -> (w130:T2)
            n46 = Unbundle By Name(w130) -> ("Y"=w131:T3)
            n47 = call "Zaber-move-1-axis-v2.vi"("Lockstep?"=w134, "Wait to complete"=w133, "Movement Type"=enum16{"relative", "absolute"}."relative", "error in"=w126, "Zaber parameters"=w131, "Port In"=w127) -> ("error out"=w125:errorcluster)  [unwired: 3 in, 2 out]
          }
          event "X Abs": Value Change {
            w148 = FALSE  # Wait to complete
            w149 = FALSE  # Lockstep?
            n48 = event-data() -> ()  [unwired: 1 in, 1 out]
            n49 = Unbundle By Name(w143) -> ("Zaber Com"=w142:refnum<visa-resource-name>)
            n50 = Bundle By Name(cluster=w144, "X.Move (units)"=w141, "X.Speed (units/s)"=w138) -> (w145:T2)
            n51 = Unbundle By Name(w145) -> ("X"=w146:T3)
            n52 = call "Zaber-move-1-axis-v2.vi"("Lockstep?"=w149, "Wait to complete"=w148, "Movement Type"=enum16{"relative", "absolute"}."absolute", "error in"=w140, "Zaber parameters"=w146, "Port In"=w142) -> ("error out"=w139:errorcluster)  [unwired: 3 in, 2 out]
          }
          event "Y Abs": Value Change {
            w159 = FALSE  # Wait to complete
            w160 = TRUE  # Lockstep?
            n53 = event-data() -> ()  [unwired: 1 in, 1 out]
            n54 = Unbundle By Name(w154) -> ("Zaber Com"=w153:refnum<visa-resource-name>)
            n55 = Bundle By Name(cluster=w155, "Y.Move (units)"=w150) -> (w156:T2)
            n56 = Unbundle By Name(w156) -> ("Y"=w157:T3)
            n57 = call "Zaber-move-1-axis-v2.vi"("Lockstep?"=w160, "Wait to complete"=w159, "Movement Type"=enum16{"relative", "absolute"}."absolute", "error in"=w152, "Zaber parameters"=w157, "Port In"=w153) -> ("error out"=w151:errorcluster)  [unwired: 3 in, 2 out]
          }
          event "X Home": Value Change {
            n58 = event-data() -> ()  [unwired: 1 in, 6 out]
            n59 = Unbundle By Name(w164) -> ("Zaber Com"=w165:refnum<visa-resource-name>)
            n60 = Unbundle By Name(w163) -> ("X"=w166:T3)
            n61 = call "Zaber-home-v2.vi"("Lockstep?"=FALSE, "error in"=w162, "Zaber parameters"=w166, "Com Port"=w165) -> ("error out"=w161:errorcluster)  [unwired: 5 in, 2 out]
          }
          event "Y Home": Value Change {
            n62 = event-data() -> ()  [unwired: 1 in, 6 out]
            n63 = Unbundle By Name(w171) -> ("Zaber Com"=w172:refnum<visa-resource-name>)
            n64 = Unbundle By Name(w170) -> ("Y"=w173:T3)
            n65 = call "Zaber-home-v2.vi"("Lockstep?"=TRUE, "error in"=w169, "Zaber parameters"=w173, "Com Port"=w172) -> ("error out"=w168:errorcluster)  [unwired: 5 in, 2 out]
          }
          event "Stop": Value Change {
            n66 = event-data() -> ()  [unwired: 1 in, 6 out]
            n67 = Unbundle By Name(w184) -> ("Zaber Com"=w183:refnum<visa-resource-name>)
            n68 = Unbundle By Name(w178) -> ("X.Device (dev axis)"=w177:string, "Y.Lockstep Group (1)"=w176:u8, "Y.Device (dev axis)"=w175:string)
            n69 = call <instrlib>:"Stop.vi"("error in (no error)"=w181, "Device and Axis"=w177, "VISA resource name"=w183) -> ("error out"=w180:errorcluster, "VISA resource name out"=w182:refnum<visa-resource-name>)  [unwired: 7 in]
            n70 = call <instrlib>:"Lockstep Stop.vi"("error in (no error)"=w180, "Device Number"=w175, "Lockstep Group (1)"=w176, "VISA resource name"=w182) -> ("error out"=w179:errorcluster)  [unwired: 6 in, 1 out]
          }
          event "Request": Value Change {
            n71 = event-data() -> ()  [unwired: 1 in, 6 out]
            n72 = Unbundle By Name(w187) -> ("MCU Com"=w186:refnum<visa-resource-name>)
            n73 = call "AR-Interlock-monitor-v2.vi"("Action"=AR-Interlock-monitor-comands."Request", "error in"=w189, "Inlk Com"=w186) -> ("error out"=w188:errorcluster, "Intlk Data"=w190:T12, "Raw Output"=w191:string)  [unwired: 4 in, 2 out]
            n74 = local write "Gating Data"(w190) -> ()
            n75 = local write "MCU Gating Raw Output"(w191) -> ()
          }
          event "Clear": Value Change {
            n76 = event-data() -> ()  [unwired: 1 in, 6 out]
            n77 = Unbundle By Name(w199) -> ("MCU Com"=w195:refnum<visa-resource-name>)
            n78 = call "AR-Interlock-monitor-v2.vi"("Action"=AR-Interlock-monitor-comands."Clear Data" ("t"), "error in"=w200, "Inlk Com"=w195) -> ("error out"=w197:errorcluster, "Raw Output"=w192:string)  [unwired: 4 in, 3 out]
            n79 = local write "MCU Gating Raw Output"(w192) -> ()
            n80 = call "AR-Interlock-monitor-v2.vi"("Action"=AR-Interlock-monitor-comands."Request", "error in"=w197, "Inlk Com"=w195) -> ("error out"=w196:errorcluster, "Intlk Data"=w193:T12)  [unwired: 4 in, 3 out]
            n81 = local write "Gating Data"(w193) -> ()
          }
        }
      }
    }
    n82 = call "Stop-FGV.vi"("Action (RD)"=enum16{"Init", "WR", "RD"}."RD", "error in"=w36) -> ("error out"=w34:errorcluster, "Out"=w35:bool)  [unwired: 8 in]
    n83 = Or(x=w35, y=w34) -> (x .or. y?=w40:bool)
  }
  n84 = while {
    tunnel: w18 -> [w209]
    tunnel: [w201] -> w16
    stop <- w212 stop-if-true
    # "Run Script trigger"
    n85 = local read "Axis params"() -> (w205:T2)
    n86 = local read "Instr Refs"() -> (w206:T15)
    n87 = Wait (ms)(milliseconds to wait=u32 10) -> ()  [unwired: 1 out]
    n88 = for {
      tunnel: "Script" -> [w515] mode=indexing
      tunnel: [w514] -> w204 mode=indexing
      n89 = Unbundle By Name(w515) -> ("Step#"=w514:dbl)
    }
    n90 = call "AR-msg-vars-FGV.vi"("Action"=enum16{"Init", "WR", "RD"}."RD") -> ("msg-var"=w208:T1)  [unwired: 9 in, 1 out]
    n91 = Unbundle By Name(w208) -> ("Run Rcp"=w203:bool)
    n92 = case shown="True" w203 {
      tunnel: w204 -> [_ w222]
      tunnel: "Script" -> [_ w221]
      tunnel: w209 -> [w214 w220]
      tunnel: w206 -> [_ w219]
      tunnel: w205 -> [_ w218]
      tunnel: [w214 w217] -> w201
      frame False {
        n93 = property on="Stop" class="Bool"("DisabledEnum"=T19."Disabled and Grayed Out" ("Disabled")) -> ()  [unwired: 2 in, 2 out]
      }
      frame True {
        w216 = 0
        # "Run Sequence"
        n94 = while {
          tunnel: w221 -> [w226]
          tunnel: w222 -> [w253]
          shift-right: [w251] -> _
          shift-left: w216 -> [w227]
          shift-right: [w248] -> _
          shift-left: w216 -> [w252]
          tunnel: w219 -> [w233]
          tunnel: w218 -> [w240]
          shift-right: [w238] -> w217
          shift-left: w220 -> [w235]
          shift-right: [w228] -> _
          shift-left: w216 -> [w229]
          stop <- w241 stop-if-true
          # ">wait cntr>"
          # "Step through\ncontrol event handle"
          # ">Dev refs>"
          # ">axis param>"
          # "Use -1 index for command array\nif need to quit loop prematuraly.\n-1 will go to default case \"End\""
          # ">loop cntr>"
          # ">prgm cntr>"
          n95 = case shown="True" "Step" {
            tunnel: w235 -> [w255 w256]
            tunnel: [w255 w256] -> w234
            frame False {
            }
            frame True {
              n96 = while {
                stop <- w257 stop-if-true
                n97 = event shown="[1] \"Next\": Value Change" {
                  selector: _ -> [_ _]
                  dyn-events: _ -> [_ _]
                  timeout: 100 -> [_ _]
                  tunnel: [_ "Next"] -> w257
                  event Timeout {
                    n98 = event-data() -> ()  [unwired: 1 in, 3 out]
                  }
                  event "Next": Value Change {
                    n99 = event-data() -> ()  [unwired: 1 in, 3 out]
                  }
                }
              }
            }
          }
          n100 = Index Array(array=w226, index=w227) -> (element=w225:T7)
          "Next command" <- w225
          n101 = Unbundle By Name(w225) -> ("Commands"=w230:T8, "Parameter1"=w254:dbl, "Parameter2"=w250:dbl, "Parameter3"=w237:dbl)  [unwired: 1 out]
          n102 = local read "Simulate Laser"() -> (w224:bool)
          n103 = Increment(x=w227) -> (x+1=w249:i32)
          n104 = case shown="\"End\", Default" w230 {
            tunnel: w254 -> [_ _ _ w312 w333 w354 w374 _ w409 w445 w477 w498 _]
            tunnel: w253 -> [_ _ _ _ _ _ _ _ _ _ w478 _ _]
            tunnel: w252 -> [w274 w287 w300 w321 w342 w363 w383 w393 w415 w451 w476 w506 w513]
            tunnel: [w275 w288 w301 w322 w343 w364 w384 w392 w414 w450 w472 w507 w512] -> w251
            tunnel: w250 -> [_ _ _ w311 w332 w353 w373 _ _ _ w475 _ _]
            tunnel: w249 -> [w275 w288 w301 w322 w343 w364 w384 w392 w414 w450 w474 w509 w512]
            tunnel: [w274 w287 w300 w321 w342 w363 w383 w393 w415 w451 w468 w506 w513] -> w248
            tunnel: [w260 w277 w289 w303 w325 w345 w365 _ w395 w431 _ w479 TRUE] -> w244
            tunnel: w234 -> [w273 w286 w299 w319 w340 w361 w381 w386 w412 w448 w466 w499 w510]
            tunnel: w233 -> [w271 w283 w296 w315 w336 w357 w377 w387 w413 w449 _ w505 _]
            tunnel: w240 -> [w268 w284 w297 w313 w334 w355 w375 _ _ _ _ w503 _]
            tunnel: [w261 w276 w291 w305 w323 w347 w367 w386 w396 w432 w466 w481 w510] -> w238
            tunnel: [w262 w278 w290 w304 w326 w346 w366 _ w404 w441 _ w480 _] -> w239
            tunnel: w237 -> [_ _ _ w310 w331 w352 w372 _ _ _ _ _ _]
            tunnel: w229 -> [_ _ _ _ _ _ _ _ _ _ _ w492 _]
            tunnel: [_ _ _ _ _ _ _ _ _ _ _ w489 _] -> w228
            tunnel: w224 -> [_ _ _ _ _ _ _ _ w394 w430 _ _ _]
            tunnel: "Accel Ena" -> [_ _ _ w302 w324 _ _ _ _ _ _ _ _]
            frame "Home All" {
              n105 = Unbundle By Name(w271) -> ("Zaber Com"=w266:refnum<visa-resource-name>)
              n106 = Unbundle By Name(w268) -> ("Y"=w267:T3)
              n107 = Unbundle By Name(w268) -> ("X"=w270:T3)
              n108 = call "Zaber-home-v2.vi"("Lockstep?"=FALSE, "error in"=w273, "Zaber parameters"=w270, "Com Port"=w266) -> ("error out"=w269:errorcluster)  [unwired: 5 in, 2 out]
              n109 = call "Zaber-home-v2.vi"("Lockstep?"=TRUE, "error in"=w269, "Zaber parameters"=w267, "Com Port"=w266) -> ("error out"=w261:errorcluster)  [unwired: 5 in, 2 out]
              n110 = Unbundle By Name(w261) -> ("status"=w260:bool)
              n111 = Select(t="Zaber", s=w260, f="") -> (s? t:f=w262:string)
            }
            frame "X Home" {
              n112 = Unbundle By Name(w283) -> ("Zaber Com"=w281:refnum<visa-resource-name>)
              n113 = Unbundle By Name(w284) -> ("X"=w282:T3)
              n114 = call "Zaber-home-v2.vi"("Lockstep?"=FALSE, "error in"=w286, "Zaber parameters"=w282, "Com Port"=w281) -> ("error out"=w276:errorcluster)  [unwired: 5 in, 2 out]
              n115 = Unbundle By Name(w276) -> ("status"=w277:bool)
              n116 = Select(t="Zaber", s=w277, f="") -> (s? t:f=w278:string)
            }
            frame "Y Home" {
              n117 = Unbundle By Name(w296) -> ("Zaber Com"=w294:refnum<visa-resource-name>)
              n118 = Unbundle By Name(w297) -> ("Y"=w295:T3)
              n119 = call "Zaber-home-v2.vi"("Lockstep?"=TRUE, "error in"=w299, "Zaber parameters"=w295, "Com Port"=w294) -> ("error out"=w291:errorcluster)  [unwired: 5 in, 2 out]
              n120 = Unbundle By Name(w291) -> ("status"=w289:bool)
              n121 = Select(t="Zaber", s=w289, f="") -> (s? t:f=w290:string)
            }
            frame "X Move Rel" {
              w317 = FALSE  # Wait to complete
              w318 = FALSE  # Lockstep?
              n122 = local write "Accel Activ"(w302) -> ()
              n123 = Bundle By Name(cluster=w313, "X.Move (units)"=w312, "X.Direction(-1,1)"=w311, "X.Speed (units/s)"=w310) -> (w309:T2)
              n124 = Unbundle By Name(w315) -> ("Zaber Com"=w314:refnum<visa-resource-name>)
              n125 = Unbundle By Name(w309) -> ("X"=w308:T3)
              n126 = call "Zaber-move-1-axis-v2.vi"("Lockstep?"=w318, "Wait to complete"=w317, "Movement Type"=enum16{"relative", "absolute"}."relative", "error in"=w319, "Zaber parameters"=w308, "Port In"=w314) -> ("error out"=w305:errorcluster)  [unwired: 3 in, 2 out]
              n127 = Unbundle By Name(w305) -> ("status"=w303:bool)
              n128 = Select(t="Zaber", s=w303, f="") -> (s? t:f=w304:string)
              n129 = Wait (ms)(milliseconds to wait=u32 1) -> ()  [unwired: 1 out]
            }
            frame "X Move Abs" {
              w338 = FALSE  # Wait to complete
              w339 = FALSE  # Lockstep?
              n130 = local write "Accel Activ"(w324) -> ()
              n131 = Bundle By Name(cluster=w334, "X.Move (units)"=w333, "X.Direction(-1,1)"=w332, "X.Speed (units/s)"=w331) -> (w330:T2)
              n132 = Unbundle By Name(w336) -> ("Zaber Com"=w335:refnum<visa-resource-name>)
              n133 = Unbundle By Name(w330) -> ("X"=w329:T3)
              n134 = call "Zaber-move-1-axis-v2.vi"("Lockstep?"=w339, "Wait to complete"=w338, "Movement Type"=enum16{"relative", "absolute"}."absolute", "error in"=w340, "Zaber parameters"=w329, "Port In"=w335) -> ("error out"=w323:errorcluster)  [unwired: 3 in, 2 out]
              n135 = Unbundle By Name(w323) -> ("status"=w325:bool)
              n136 = Select(t="Zaber", s=w325, f="") -> (s? t:f=w326:string)
              n137 = flat-sequence {
                tunnel: w323 -> [_]
                frame #0 {
                  n138 = local write "Accel Activ"(FALSE ("Accel Activ")) -> ()
                }
              }
              n139 = Wait (ms)(milliseconds to wait=u32 1) -> ()  [unwired: 1 out]
            }
            frame "Y Move Rel" {
              w359 = FALSE  # Wait to complete
              w360 = TRUE  # Lockstep?
              n140 = Bundle By Name(cluster=w355, "Y.Move (units)"=w354, "Y.Direction(-1,1)"=w353, "Y.Speed (units/s)"=w352) -> (w351:T2)
              n141 = Unbundle By Name(w357) -> ("Zaber Com"=w356:refnum<visa-resource-name>)
              n142 = Unbundle By Name(w351) -> ("Y"=w350:T3)
              n143 = call "Zaber-move-1-axis-v2.vi"("Lockstep?"=w360, "Wait to complete"=w359, "Movement Type"=enum16{"relative", "absolute"}."relative", "error in"=w361, "Zaber parameters"=w350, "Port In"=w356) -> ("error out"=w347:errorcluster)  [unwired: 3 in, 2 out]
              n144 = Unbundle By Name(w347) -> ("status"=w345:bool)
              n145 = Select(t="Zaber", s=w345, f="") -> (s? t:f=w346:string)
              n146 = Wait (ms)(milliseconds to wait=u32 100) -> ()  [unwired: 1 out]
            }
            frame "Y Move Abs" {
              w379 = FALSE  # Wait to complete
              w380 = TRUE  # Lockstep?
              n147 = Bundle By Name(cluster=w375, "Y.Move (units)"=w374, "Y.Direction(-1,1)"=w373, "Y.Speed (units/s)"=w372) -> (w371:T2)
              n148 = Unbundle By Name(w377) -> ("Zaber Com"=w376:refnum<visa-resource-name>)
              n149 = Unbundle By Name(w371) -> ("Y"=w370:T3)
              n150 = call "Zaber-move-1-axis-v2.vi"("Lockstep?"=w380, "Wait to complete"=w379, "Movement Type"=enum16{"relative", "absolute"}."absolute", "error in"=w381, "Zaber parameters"=w370, "Port In"=w376) -> ("error out"=w367:errorcluster)  [unwired: 3 in, 2 out]
              n151 = Unbundle By Name(w367) -> ("status"=w365:bool)
              n152 = Select(t="Zaber", s=w365, f="") -> (s? t:f=w366:string)
              n153 = Wait (ms)(milliseconds to wait=u32 100) -> ()  [unwired: 1 out]
            }
            frame "Reset Intlk Timer" {
              n154 = Unbundle By Name(w387) -> ("MCU Com"=w385:refnum<visa-resource-name>)
              n155 = call "AR-Interlock-monitor-v2.vi"("Action"=AR-Interlock-monitor-comands."Clear Data", "error in"=w386, "Inlk Com"=w385) -> ("error out"=w390:errorcluster)  [unwired: 4 in, 4 out]
              n156 = call "AR-Interlock-monitor-v2.vi"("Action"=AR-Interlock-monitor-comands."Request", "error in"=w390, "Inlk Com"=w385) -> ("error out"=w391:errorcluster)  [unwired: 4 in, 4 out]
              n157 = call <vilib>:"Clear Errors.vi"("error in (no error)"=w391) -> ()  [unwired: 5 in, 2 out]
            }
            frame "Laser Sys ON" {
              n158 = Equal?(x=w409, y=1.0) -> (x = y?=w400:bool)
              n159 = Unbundle By Name(w413) -> ("LaserSysRef Out"=w411:refnum<k24>, "LaserControl Ref Out"=w410:refnum<k24>)
              n160 = Select(t=nLight-wait-states."Wait SysON" ("Action"), s=w400, f=nLight-wait-states."Wait SysOFF" ("Action")) -> (s? t:f=w397:T20)
              n161 = call "nLight-SystemON-ENA.vi"("ENA"=FALSE, "SysON"=w400, "Simulate (F)"=w394, "error in"=w412, "LaserControl Ref"=w410, "LaserSysRef"=w411) -> ("error out"=w403:errorcluster, "LaserControl Ref Out"=w402:refnum<k24>, "LaserSysRef Out"=w401:refnum<k24>)  [unwired: 3 in]
              n162 = disable-structure shown="Enabled" {
                disable-tunnel: w403 -> [w425 w428]
                disable-tunnel: w402 -> [w424 _]
                disable-tunnel: w401 -> [w423 _]
                disable-tunnel: w397 -> [w422 _]
                disable-tunnel: [w418 w427] -> w396
                disable-tunnel: [w417 FALSE] -> w395
                disable-tunnel: w394 -> [w416 _]
                frame Disabled {
                  n163 = call "nLight-Wait-for-Status.vi"("Timeout (s)"=5.0, "Action"=w422, "error in"=w425, "Simulate (F)"=w416, "LaserControl Ref"=w424, "LaserSysRef"=w423) -> ("error out"=w418:errorcluster, "Error"=w420:bool, "Fault"=w419:bool)  [unwired: 3 out]
                  n164 = Compound Arithmetic op=OR(w419, w420, w418) -> (w417:bool)
                }
                frame Enabled {
                  n165 = call "Sys on"("error in (no error)"=w428, "Delay Time (s)"=5.0) -> ("error out"=w427:errorcluster)  [unwired: 9 in]
                }
              }
              n166 = Select(t="Laser", s=w395, f="") -> (s? t:f=w404:string)
            }
            frame "Laser ENA" {
              n167 = Equal?(x=w445, y=1.0) -> (x = y?=w434:bool)
              n168 = Unbundle By Name(w449) -> ("LaserSysRef Out"=w447:refnum<k24>, "LaserControl Ref Out"=w446:refnum<k24>)
              n169 = Select(t=nLight-wait-states."Wait ENA" ("Action"), s=w434, f=nLight-wait-states."Wait DIS" ("Action")) -> (s? t:f=w435:T20)
              n170 = call "nLight-SystemON-ENA.vi"("ENA"=w434, "SysON"=TRUE, "Simulate (F)"=w430, "error in"=w448, "LaserControl Ref"=w446, "LaserSysRef"=w447) -> ("error out"=w440:errorcluster, "LaserControl Ref Out"=w439:refnum<k24>, "LaserSysRef Out"=w438:refnum<k24>)  [unwired: 3 in]
              n171 = disable-structure shown="Enabled" {
                disable-tunnel: w440 -> [w461 w464]
                disable-tunnel: w439 -> [w460 _]
                disable-tunnel: w438 -> [w459 _]
                disable-tunnel: w435 -> [w458 _]
                disable-tunnel: [w454 w463] -> w432
                disable-tunnel: [w453 FALSE] -> w431
                disable-tunnel: w430 -> [w452 _]
                frame Disabled {
                  n172 = call "nLight-Wait-for-Status.vi"("Timeout (s)"=5.0, "Action"=w458, "error in"=w461, "Simulate (F)"=w452, "LaserControl Ref"=w460, "LaserSysRef"=w459) -> ("error out"=w454:errorcluster, "Error"=w456:bool, "Fault"=w455:bool)  [unwired: 3 out]
                  n173 = Compound Arithmetic op=OR(w455, w456, w454) -> (w453:bool)
                }
                frame Enabled {
                  n174 = call "ENA delay"("error in (no error)"=w464, "Delay Time (s)"=5.0) -> ("error out"=w463:errorcluster)  [unwired: 9 in]
                }
              }
              n175 = Select(t="Laser", s=w431, f="") -> (s? t:f=w441:string)
            }
            frame "Repeat" {
              n176 = Search 1D Array(1D array=w478, element=w477) -> (index of element=w473:i32)  [unwired: 1 in]
              n177 = Increment(x=w476) -> (x+1=w470:i32)
              n178 = Less Or Equal?(x=w475, y=w470) -> (x <= y?=w471:bool)
              n179 = Select(t=w474, s=w471, f=w473) -> (s? t:f=w472:i32)
              n180 = Select(t=0, s=w471, f=w470) -> (s? t:f=w468:i32)
              n181 = Wait (ms)(milliseconds to wait=u32 100) -> ()  [unwired: 1 out]
            }
            frame "Wait" {
              # "Wait is implemented by looping through the same Wait state\n(doesn't increment the \"prgm cntr\" untill Timer expires."
              # "Properly reset timer\nthe first time it enters \nthe wait state"
              # "Update pos/speed\ngraph"
              n182 = Unbundle By Name(w503) -> ("X.Microstep Size"=w502:dbl, "X.Device (dev axis)"=w501:string, "X.Units"=w500:T9)
              n183 = Unbundle By Name(w505) -> ("Zaber Com"=w504:refnum<visa-resource-name>)
              n184 = call <instrlib>:"Read Current Position.vi"("Units (0: microsteps)"=w500, "error in (no error)"=w499, "Device and Axis"=w501, "Microstep Size (0)"=w502, "VISA resource name"=w504) -> ("error out"=w481:errorcluster, "Position"=w488:dbl)  [unwired: 4 in, 1 out]
              n185 = local write "X Position"(w488) -> ()
              n186 = Unbundle By Name(w481) -> ("status"=w479:bool)
              n187 = Equal To 0?(x=w492) -> (x = 0?=w497:bool)
              n188 = Select(t=enum16{"Reset", "Start"}."Reset" ("Action"), s=w497, f=enum16{"Reset", "Start"}."Start") -> (s? t:f=w495:enum16{"Reset", "Start"})
              n189 = Increment(x=w492) -> (x+1=w491:i32)
              n190 = Select(t="Zaber", s=w479, f="") -> (s? t:f=w480:string)
              n191 = call "Elapsed-Timer.vi"("Action"=w495, "Target (mS)"=w498) -> ("Time Elapsed"=w493:bool, "Loop time (ms)"=w487:u32)  [unwired: 7 in, 1 out]
              n192 = call "AR-Build-Axis-position-speed-graph.vi"("Select"="Select", "Action"=enum16{"Init", "WR", "RD"}."WR", "Loop time"=w487, "X Pos"=w488) -> ("Pos/Speed"=→"X Axis Pos/Speed":cluster{u32[], dbl[]})  [unwired: 7 in]
              n193 = Select(t=0, s=w493, f=w491) -> (s? t:f=w489:i32)
              n194 = Decrement(x=w509) -> (x-1=w508:i32)
              n195 = Select(t=w509, s=w493, f=w508) -> (s? t:f=w507:i32)
            }
            frame "End", Default {
            }
          }
          n196 = call "Stop-FGV.vi"("Action (RD)"=enum16{"Init", "WR", "RD"}."RD") -> ("Out"=w245:bool)  [unwired: 9 in, 1 out]
          n197 = Compound Arithmetic op=OR(w244, w245, "Stop") -> (w241:bool)
          n198 = Not(x=w241) -> (.not. x?=w243:bool)
          n199 = local read "msg-var"() -> (w232:T1)
          n200 = Bundle By Name(cluster=w232, "Run Rcp"=w243, "Rcp Stopped"=w241, "Err Device"=w239) -> (w231:T1)
          n201 = call "AR-msg-vars-FGV.vi"("Action"=enum16{"Init", "WR", "RD"}."WR", "msg-var in"=w231) -> ()  [unwired: 8 in, 2 out]
        }
        n202 = property on="Stop" class="Bool"("DisabledEnum"=T19."Enabled" ("Disabled")) -> ()  [unwired: 2 in, 2 out]
      }
    }
    n203 = call "Stop-FGV.vi"("Action (RD)"=enum16{"Init", "WR", "RD"}."RD") -> ("Out"=w212:bool)  [unwired: 9 in, 1 out]
  }
  n204 = local read "Simulate Laser"() -> (w6:bool)
  n205 = while {
    shift-right: [w529] -> w10
    shift-left: w1 -> [w530]
    shift-right: [w527] -> _
    shift-left: "Init" ("Action") -> [w524]
    shift-right: [w522] -> _
    shift-left: T15 {"Zaber Com"="", "MCU Com"="", "LaserSysRef Out"=refnum, "LaserControl Ref Out"=refnum} ("Instr Refs") -> [w523]
    shift-right: [w518] -> _
    shift-left: T2 {"X"={"Device (dev axis)"="1 3", "Lockstep Group (1)"=1, "Units"=enum."millimeters", "Microstep Size"=4.21875, "Move (units)"=0.0, "Direction(-1,1)"=1, "Speed (units/s)"=1500.0}, "Y"={"Device (dev axis)"="1", "Lockstep Group (1)"=1, "Units"=enum."millimeters", "Microstep Size"=0.496094, "Move (units)"=0.0, "Direction(-1,1)"=1, "Speed (units/s)"=45.0}} ("Axis params") -> [w521]
    tunnel: w22 -> [w520]
    tunnel: w6 -> [w517]
    stop <- w525 stop-if-true
    # ">Dev refs>"
    # ">axis param>"
    n206 = Wait (ms)(milliseconds to wait=u32 10) -> ()  [unwired: 1 out]
    n207 = case shown="\"Init\", Default" w524 {
      selector: w524 -> [_ _ w627 _ w668 _ w849]
      tunnel: [w542 w601 w626 w649 w669 w815 w836] -> w529
      tunnel: w530 -> [w545 w620 w637 w647 w670 w812 w844]
      tunnel: [w538 w597 w623 w652 w671 "Commands" ("Action") w849] -> w526
      tunnel: [_ _ _ _ _ _ w847] -> w525
      tunnel: w523 -> [w544 w611 w639 w651 w665 w806 w840]
      tunnel: [w543 w611 w639 w651 w665 w806 w840] -> w522
      tunnel: ["Axis params" w619 w640 w650 w666 w814 w846] -> w518
      tunnel: w521 -> [_ w619 w640 w650 w667 w814 w846]
      tunnel: w520 -> [w537 _ _ _ _ _ _]
      tunnel: "Recipe (csv)" -> [w541 _ _ _ w664 _ _]
      tunnel: w517 -> [w532 w608 _ _ w663 w803 w833]
      frame "Init", Default {
        n208 = event shown="[0] \"Init\": Value Change" {
          selector: _ -> [_ _]
          dyn-events: _ -> [_ _]
          timeout: 100 -> [_ _]
          tunnel: w545 -> [w563 w595]
          tunnel: [w584 w590] -> w534
          tunnel: [w564 w595] -> w542
          tunnel: w541 -> [w561 _]
          tunnel: "Com ports" -> [w583 w592]
          tunnel: [w578 "Init" ("f")] -> w538
          tunnel: w537 -> [w577 _]
          tunnel: [w568 w591] -> w533
          tunnel: [w557 _] -> w536
          tunnel: [w558 _] -> w535
          tunnel: w532 -> [w556 _]
          tunnel: "Axis params" -> [w551 _]
          event "Init": Value Change {
            w555 = TRUE  # Wait to complete
            w546 = TRUE  # Lockstep?
            # "Some housekeeping"
            n209 = event-data() -> ()  [unwired: 1 in, 6 out]
            n210 = Unbundle By Name(w583) -> ("Zaber Com"=w584:refnum<visa-resource-name>, "Laser IP"=w576:string, "MCU Com"=w568:refnum<visa-resource-name>)
            n211 = Bundle By Name(cluster=w551, "Y.Move (units)"="Start Y Position") -> (w549:T2)
            n212 = call "Read-exec-script.vi"("error in"=w563, "file (use dialog)"=w561) -> ("error out"=w562:errorcluster, "Commands"=w560:T7[])  [unwired: 7 in, 1 out]
            n213 = local write "Script"(w560) -> ()
            n214 = for {
              tunnel: w577 -> [w587] mode=indexing
              n215 = property class="Page"(reference=w587, "PageEnb"=T17."Page Enabled" ("Page Enabled State")) -> ()  [unwired: 1 in, 2 out]
            }
            n216 = call <vilib>:"Clear Errors.vi"("error in (no error)"=w562) -> ("error out"=w575:errorcluster)  [unwired: 5 in, 1 out]
            n217 = call "nLight-Connect-Clear.vi"("Simulate?"=w556, "error in"=w575, "targetIpAddress"=w576) -> ("error out"=w559:errorcluster, "IsConnected"=w569:bool, "LaserControl Ref Out"=w558:refnum<k24>, "LaserSysRef Out"=w557:refnum<k24>)  [unwired: 5 in]
            "Laser OK" <- w569
            n218 = call "AR-Interlock-monitor-v2.vi"("Action"=AR-Interlock-monitor-comands."Init", "error in"=w575, "Inlk Com"=w568) -> ("error out"=w571:errorcluster)  [unwired: 4 in, 4 out]
            n219 = Unbundle By Name(w549) -> ("Y"=w548:T3)
            n220 = call "Zaber-multi-init.vi"("Log @"="At init stage", "error in (no error)"=w575, "Port #"=w584) -> ("error IO"=w553:errorcluster, "Port Out"=w550:refnum<visa-resource-name>, "Port OK"=w582:bool)  [unwired: 3 in, 3 out]
            "Zaber OK" <- w582
            n221 = call "Zaber-move-1-axis-v2.vi"("Lockstep?"=w546, "Wait to complete"=w555, "Movement Type"=enum16{"relative", "absolute"}."absolute", "error in"=w553, "Zaber parameters"=w548, "Port In"=w550) -> ("error out"=w552:errorcluster)  [unwired: 3 in, 2 out]
            n222 = property on="Init" class="Bool"("DisabledEnum"=T19."Disabled" ("Disabled")) -> (error out=w566:errorcluster)  [unwired: 2 in, 1 out]
            n223 = property on="Quit" class="Bool"(error in=w566, "DisabledEnum"=T19."Enabled" ("Disabled")) -> ()  [unwired: 1 in, 2 out]
            n224 = Select(t=FALSE, s=w571, f=TRUE) -> (s? t:f=w570:bool)
            "MCU INLK" <- w570
            n225 = Compound Arithmetic op=AND(w569, w570, w582) -> (w581:bool)
            n226 = Select(t="Enable Mon Loop" ("f"), s=w581, f="Quit") -> (s? t:f=w578:string)
            n227 = Merge Errors(w559, w571, w552) -> (w564:errorcluster)
          }
          event Timeout {
            w589 = T19."Disabled and Grayed Out" ("Disabled")
            w588 = FALSE
            n228 = event-data() -> ()  [unwired: 1 in, 1 out]
            n229 = Unbundle By Name(w592) -> ("MCU Com"=w591:refnum<visa-resource-name>, "Zaber Com"=w590:refnum<visa-resource-name>)
            n230 = local write "Mode RDY"(w588) -> ()
            n231 = property on="MCU INLK" class="Bool"("Value"=w588) -> ()  [unwired: 2 in, 2 out]
            n232 = property on="Zaber OK" class="Bool"("Value"=w588) -> ()  [unwired: 2 in, 2 out]
            n233 = property on="Quit" class="Bool"("DisabledEnum"=T19."Disabled" ("Disabled")) -> ()  [unwired: 2 in, 2 out]
            n234 = property on="Laser OK" class="Bool"("Value"=w588) -> ()  [unwired: 2 in, 2 out]
            n235 = property on="Init" class="Bool"("DisabledEnum"=T19."Enabled" ("Disabled")) -> ()  [unwired: 2 in, 2 out]
            n236 = property on="ENA" class="Bool (strict)"("DisabledEnum"=w589) -> ()  [unwired: 2 in, 2 out]
            n237 = property on="Next" class="Bool"("DisabledEnum"=w589) -> ()  [unwired: 2 in, 2 out]
            n238 = property on="EMIT!" class="Bool (strict)"("DisabledEnum"=w589) -> ()  [unwired: 2 in, 2 out]
          }
        }
        n239 = Bundle By Name(cluster=w544, "MCU Com"=w533, "Zaber Com"=w534, "LaserSysRef Out"=w536, "LaserControl Ref Out"=w535) -> (w543:T15)
      }
      frame "Enable Mon Loop" {
        w606 = 1 items=["HW", "API", "CLI", "INET, CONTROL_INT_MASK"] ("ControllingInterface")
        n240 = call "Time Delay2"("error in (no error)"=w620, "Delay Time (s)"=0.5) -> ("error out"=w614:errorcluster)  [unwired: 9 in]
        n241 = local read "msg-var"() -> (w618:T1)
        n242 = Bundle By Name(cluster=w618, "Run Axis Loop"=TRUE) -> (w617:T1)
        n243 = Unbundle By Name(w611) -> ("LaserSysRef Out"=w609:refnum<k24>, "LaserControl Ref Out"=w610:refnum<k24>)
        n244 = call "AR-msg-vars-FGV.vi"("Action"=enum16{"Init", "WR", "RD"}."WR", "error in"=w614, "msg-var in"=w617) -> ("error out"=w612:errorcluster)  [unwired: 7 in, 1 out]
        n245 = call "nLight-Check-Control-Interface.vi"("Simulate (F)"=w608, "error in"=w612, "LaserControl Ref"=w610, "LaserSysRef"=w609) -> ("error out"=w601:errorcluster, "ExternalGate"=w603:bool, "ControllingInterface"=w607:i32, "ProfileModeEnabled"=w605:bool)  [unwired: 2 in, 2 out]
        "Controll Interface" <- w607
        "External Gate" <- w603
        "Profile Mode" <- w605
        n246 = Not(x=w605) -> (.not. x?=w602:bool)
        n247 = Equal?(x=w606, y=w607) -> (x = y?=w604:bool)
        n248 = Compound Arithmetic op=AND(w604, w603, w602) -> (w600:bool)
        n249 = case shown="False" w600 {
          frame False {
            n250 = One Button Dialog(message="Laser must be configured as API(GUI) Control Interface with External Gate control.\n\nCheck the Laser configuration in nLight Application and try again.") -> ()  [unwired: 1 in, 1 out]
          }
          frame True {
          }
        }
        n251 = Select(t="Test MCU Flags" ("Action"), s=w600, f="Quit" ("Action")) -> (s? t:f=w597:string)
      }
      frame "Test MCU Flags" {
        # "Repeat if flags are not set correctly\nOnly 1 at a time"
        n252 = Unbundle By Name(w639) -> ("MCU Com"=w636:refnum<visa-resource-name>)
        n253 = call "AR-Interlock-monitor-v2.vi"("Action"=AR-Interlock-monitor-comands."Request", "error in"=w637, "Inlk Com"=w636) -> ("error out"=w626:errorcluster, "Intlk Data"=w634:T12)  [unwired: 4 in, 3 out]
        n254 = Unbundle By Name(w634) -> ("Chamber Ena"=w632:bool, "Profiler Ena"=w631:bool, "OPower Ena"=w630:bool)
        n255 = Bundle By Name(cluster=T6 {"Chamber Ena"=FALSE, "Profiler Ena"=FALSE, "OPower Ena"=FALSE} ("MCU Gating Flags"), "Chamber Ena"=w632, "Profiler Ena"=w631, "OPower Ena"=w630) -> (→"MCU Gating Flags":T6)
        n256 = Compound Arithmetic op=XOR(w632, w631, w630) -> (w628:bool)
        n257 = case shown="False" w628 {
          tunnel: [w641 TRUE ("T button?")] -> w625
          frame False {
            n258 = Two Button Dialog(message="MCU Gating Control\n\nOnly 1 flag must be enabled in order for the Laser Gate control to be active.\nSet the correct Flags and click OK.\n\nClicking on Quit will terminate the program.", 1:"Quit" ("F button name (\"Cancel\")")) -> (T button?=w641:bool)  [unwired: 1 in]
          }
          frame True {
          }
        }
        n259 = Select(t="Test Gating" ("Action"), s=w628, f=w627) -> (s? t:f=w624:string)
        n260 = Select(t=w624, s=w625, f="Quit") -> (s? t:f=w623:string)
      }
      frame "Test Gating" {
        n261 = call "Display Message to User"("error in (no error)"=w647) -> ("error out"=w646:errorcluster, "YES"=w645:bool)  [unwired: 9 in]
        n262 = case shown="True" w645 {
          tunnel: [w655 w660] -> w649
          tunnel: w646 -> [w655 w656]
          frame False {
          }
          frame True {
            n263 = local read "Com ports"() -> (w662:T5)
            n264 = call "AR-Check-Gating.vi"("error in"=w656, "Zaber parameters"="X Axis Initial Test Parameters", "Com ports"=w662) -> ("error out"=w660:errorcluster, "Timed Out"=→"Gating Timedout":bool, "Time Delta (mS)"=→"Delta Time (mS)":dbl, "X Pos Triggered"=→"X Position Triggered":dbl)  [unwired: 5 in]
          }
        }
        n265 = Select(t="Commands" ("Action"), s=TRUE, f="Quit" ("Action")) -> (s? t:f=w652:string)
      }
      frame "Commands" {
        n266 = event shown="[1] \"Run script\": Value Change" {
          selector: _ -> [_ _ _ _ _ _ _ _ _ _ _]
          dyn-events: _ -> [_ _ _ _ _ _ _ _ _ _ _]
          timeout: 100 -> [_ _ _ _ _ _ _ _ _ _ _]
          tunnel: [w686 w702 w714 w724 w739 w747 w762 w777 w794 "Test Gating" ("Action") "Quit" ("Action")] -> w671
          tunnel: w670 -> [w690 w692 w706 w720 w735 w756 w769 w776 w793 w798 w801]
          tunnel: [w690 w692 w705 w715 w730 w748 w763 w775 w782 w798 w801] -> w669
          tunnel: w668 -> [w682 w702 w714 w724 w739 w747 w762 w777 w794 _ _]
          tunnel: w667 -> [w680 w697 w708 w723 w738 w757 w770 w779 w796 w799 w800]
          tunnel: [w678 w697 w707 w723 w738 w757 w770 w779 w796 w799 w800] -> w666
          tunnel: w665 -> [_ _ w704 _ _ w755 w768 w778 w795 _ _]
          tunnel: w664 -> [_ _ _ w722 w737 _ _ _ _ _ _]
          tunnel: w663 -> [_ _ _ _ _ w745 w758 w772 w783 _ _]
          event Timeout {
            n267 = event-data() -> ()  [unwired: 1 in, 1 out]
            n268 = Bundle By Name(cluster=w680, "X.Units"="Select Units", "Y.Units"="Select Units", "X.Device (dev axis)"="X (dev axis)", "Y.Device (dev axis)"="Y (dev axis)", "X.Microstep Size"="X Microstep Size", "Y.Microstep Size"="Y Microstep Size") -> (w678:T2)
            n269 = call "AR-msg-vars-FGV.vi"("Action"=enum16{"Init", "WR", "RD"}."RD") -> ("msg-var"=w684:T1)  [unwired: 9 in, 1 out]
            "msg-var" <- w684
            n270 = Unbundle By Name(w684) -> ("Rcp Stopped"=w673:bool)
            n271 = case shown="False" w673 {
              frame False {
              }
              frame True {
                n272 = property on="Next" class="Bool"("DisabledEnum"=T19."Disabled and Grayed Out" ("Disabled")) -> ()  [unwired: 2 in, 2 out]
              }
            }
            n273 = Select(t="Safe", s=w673, f=w682) -> (s? t:f=w681:string)
            n274 = call "Stop-FGV.vi"("Action (RD)"=enum16{"Init", "WR", "RD"}."RD") -> ("Out"=w688:bool)  [unwired: 9 in, 1 out]
            n275 = Select(t="Quit", s=w688, f=w681) -> (s? t:f=w686:string)
          }
          event "Run script": Value Change {
            # "Ena Next Button\nwhen script started"
            n276 = event-data() -> ()  [unwired: 1 in, 1 out]
            n277 = local read "msg-var"() -> (w694:T1)
            n278 = Bundle By Name(cluster=w694, "Run Rcp"=TRUE, "Rcp Stopped"=FALSE ("Stop Rcp")) -> (w700:T1)
            n279 = call "AR-Build-Axis-position-speed-graph.vi"("Action"=enum16{"Init", "WR", "RD"}."Init", "error in (no error)"=w692) -> ()  [unwired: 9 in, 1 out]
            n280 = call "AR-msg-vars-FGV.vi"("Action"=enum16{"Init", "WR", "RD"}."WR", "msg-var in"=w700) -> ("error out"=w695:errorcluster)  [unwired: 8 in, 1 out]
            n281 = property on="Next" class="Bool"(error in=w695, "DisabledEnum"=T19."Enabled" ("Disabled")) -> ()  [unwired: 1 in, 2 out]
          }
          event "Zaber settings": Value Change {
            n282 = event-data() -> ()  [unwired: 1 in, 1 out]
            n283 = Unbundle By Name(w704) -> ("Zaber Com"=w703:refnum<visa-resource-name>)
            n284 = call "AR-Axis-update-parameters-GUI.vi"("error in"=w706, "Com"=w703) -> ("error out"=w705:errorcluster, "Axis"=→"Axis":string[], "Connected Devices"=→"Devices":string[], "Device Info"=→"Device Info":T10)  [unwired: 6 in]
            n285 = Bundle By Name(cluster=w708, "Y.Device (dev axis)"="1", "X.Device (dev axis)"="1 3") -> (w707:T2)
          }
          event "Load script": Value Change {
            n286 = event-data() -> ()  [unwired: 1 in, 1 out]
            n287 = Strip Path(path=w722) -> (stripped path=w721:path)  [unwired: 1 out]
            n288 = call "File Dialog"("start path"=w721, "error in"=w720) -> ("selected path"=w717:path, "cancelled"=w719:bool, "error out"=w718:errorcluster)  [unwired: 10 in, 1 out]
            n289 = case shown="False" w719 {
              tunnel: w718 -> [w728 w729]
              tunnel: w717 -> [w726 _]
              tunnel: [w727 w729] -> w716
              frame False {
                n290 = call "Read-exec-script.vi"("error in"=w728, "file (use dialog)"=w726) -> ("error out"=w727:errorcluster, "Commands"=w725:T7[])  [unwired: 7 in, 1 out]
                n291 = local write "Script"(w725) -> ()
              }
              frame True {
              }
            }
            n292 = call <vilib>:"Clear Errors.vi"("error in (no error)"=w716) -> ("error out"=w715:errorcluster)  [unwired: 5 in, 1 out]
          }
          event "Save script": Value Change {
            n293 = event-data() -> ()  [unwired: 1 in, 1 out]
            n294 = Strip Path(path=w737) -> (stripped path=w736:path)  [unwired: 1 out]
            n295 = call "File Dialog2"("start path"=w736, "error in"=w735) -> ("selected path"=w732:path, "cancelled"=w734:bool, "error out"=w733:errorcluster)  [unwired: 10 in, 1 out]
            n296 = case shown="False" w734 {
              tunnel: w733 -> [w743 w744]
              tunnel: w732 -> [w742 _]
              tunnel: [w740 w744] -> w731
              frame False {
                n297 = local read "Script"() -> (w741:T7[])
                n298 = call "Save-exec-script.vi"("error in"=w743, "Script array"=w741, "file (use dialog)"=w742) -> ("error out"=w740:errorcluster)  [unwired: 7 in, 1 out]
              }
              frame True {
              }
            }
            n299 = call <vilib>:"Clear Errors.vi"("error in (no error)"=w731) -> ("error out"=w730:errorcluster)  [unwired: 5 in, 1 out]
          }
          event "SysON": Value Change {
            w746 = T19."Disabled and Grayed Out" ("Disabled")
            w752 = FALSE  # ENA
            n300 = event-data() -> ("NewVal"=w751:bool)  [unwired: 1 in]
            n301 = Unbundle By Name(w755) -> ("LaserSysRef Out"=w754:refnum<k24>, "LaserControl Ref Out"=w753:refnum<k24>)
            n302 = call "nLight-SystemON-ENA.vi"("ENA"=w752, "SysON"=w751, "Simulate (F)"=w745, "error in"=w756, "LaserControl Ref"=w753, "LaserSysRef"=w754) -> ("error out"=w748:errorcluster)  [unwired: 3 in, 2 out]
            n303 = Select(t=T19."Enabled" ("Disabled"), s=w751, f=w746) -> (s? t:f=w749:T19)
            n304 = property on="ENA" class="Bool (strict)"("DisabledEnum"=w749) -> ()  [unwired: 2 in, 2 out]
            n305 = property on="EMIT!" class="Bool (strict)"("DisabledEnum"=w746) -> ()  [unwired: 2 in, 2 out]
          }
          event "ENA": Value Change {
            w761 = TRUE  # SysON
            n306 = event-data() -> ("NewVal"=w760:bool)  [unwired: 1 in]
            n307 = Unbundle By Name(w768) -> ("LaserSysRef Out"=w767:refnum<k24>, "LaserControl Ref Out"=w766:refnum<k24>)
            n308 = call "nLight-SystemON-ENA.vi"("ENA"=w760, "SysON"=w761, "Simulate (F)"=w758, "error in"=w769, "LaserControl Ref"=w766, "LaserSysRef"=w767) -> ("error out"=w763:errorcluster)  [unwired: 3 in, 2 out]
            n309 = Select(t=T19."Enabled" ("Disabled"), s=w760, f=T19."Disabled and Grayed Out" ("Disabled")) -> (s? t:f=w759:T19)
            n310 = property on="EMIT!" class="Bool (strict)"("DisabledEnum"=w759) -> ()  [unwired: 2 in, 2 out]
          }
          event "EMIT!": Value Change {
            n311 = event-data() -> ("NewVal"=w771:bool)  [unwired: 1 in]
            n312 = Unbundle By Name(w778) -> ("LaserSysRef Out"=w774:refnum<k24>, "LaserControl Ref Out"=w773:refnum<k24>)
            n313 = call "nLight-Emit.vi"("Emit!"=w771, "Simulate (F)"=w772, "error in"=w776, "LaserControl Ref"=w773, "LaserSysRef"=w774) -> ("error out"=w775:errorcluster)  [unwired: 4 in, 2 out]
          }
          event "Set Laser Params": Value Change {
            n314 = event-data() -> ()  [unwired: 1 in, 1 out]
            n315 = Unbundle By Name(w795) -> ("LaserSysRef Out"=w792:refnum<k24>, "LaserControl Ref Out"=w791:refnum<k24>)
            n316 = call "nLight-Set-Laser-Params.vi"("Simulate (F)"=w783, "Laser Params"="Laser Params", "error in"=w793, "LaserControl Ref"=w791, "LaserSysRef"=w792) -> ("error out"=w786:errorcluster, "Comanded Params"=w789:T13, "LaserControl Ref Out"=w784:refnum<k24>, "LaserSysRef Out"=w785:refnum<k24>)  [unwired: 3 in]
            n317 = Unbundle By Name(w789) -> ("Power(W)"=→"Laser Power (W)":dbl, "Duty(%)"=→"Laser Duty (%)":dbl)
            n318 = call "nLight-Beam-Profile-Mode-SubVI.vi"("Simulate (F)"=w783, "error in"=w786, "Beam-profile(0-6)"="Beam-profile(0-6)", "LaserControl Ref"=w784, "LaserSysRef"=w785) -> ("error out"=w782:errorcluster, "Ready"=→"Mode RDY":bool)  [unwired: 2 in, 3 out]
          }
          event "Re-test gating": Value Change {
            n319 = event-data() -> ()  [unwired: 1 in, 1 out]
          }
          event "Quit": Value Change {
            n320 = event-data() -> ()  [unwired: 1 in, 1 out]
          }
        }
      }
      frame "Safe" {
        # "The Script execution has been stopped by the user"
        n321 = call "AR-msg-vars-FGV.vi"("Action"=enum16{"Init", "WR", "RD"}."RD", "error in"=w812) -> ("error out"=w810:errorcluster, "msg-var"=w811:T1)  [unwired: 8 in]
        n322 = Unbundle By Name(w806) -> ("LaserSysRef Out"=w805:refnum<k24>, "LaserControl Ref Out"=w804:refnum<k24>)
        n323 = Unbundle By Name(w811) -> ("Err Device"=w809:string)
        n324 = case shown="\"Zaber\", Default" w809 {
          tunnel: w810 -> [w828 w829]
          tunnel: [w823 w829] -> w808
          tunnel: w805 -> [w827 _]
          tunnel: w804 -> [w826 _]
          tunnel: w803 -> [w821 _]
          frame "Zaber", Default {
            w825 = FALSE ("SysON")
            # "If Zaber Err OR no Err, do Lase Safe Routine"
            n325 = call "nLight-SystemON-ENA.vi"("ENA"=w825, "SysON"=w825, "Simulate (F)"=w821, "error in"=w828, "LaserControl Ref"=w826, "LaserSysRef"=w827) -> ("error out"=w824:errorcluster)  [unwired: 3 in, 2 out]
            n326 = call "Time Delay"("error in (no error)"=w824, "Delay Time (s)"=2.0) -> ("error out"=w823:errorcluster)  [unwired: 9 in]
          }
          frame "Laser" {
            # "If Laser Err show warning Msg here, no Laser Safe routine"
            n327 = One Button Dialog(message="Laser Error") -> ()  [unwired: 1 in, 1 out]
          }
        }
        n328 = local read "msg-var"() -> (w807:T1)
        n329 = Bundle By Name(cluster=w807, "Run Rcp"=FALSE, "Rcp Stopped"=FALSE) -> (w819:T1)
        n330 = call "AR-msg-vars-FGV.vi"("Action"=enum16{"Init", "WR", "RD"}."WR", "error in"=w808, "msg-var in"=w819) -> ("error out"=w815:errorcluster)  [unwired: 7 in, 1 out]
      }
      frame "Quit" {
        w847 = TRUE
        n331 = call "AR-msg-vars-FGV.vi"("Action"=enum16{"Init", "WR", "RD"}."RD", "error in"=w844) -> ("error out"=w832:errorcluster, "msg-var"=w843:T1)  [unwired: 8 in]
        n332 = Unbundle By Name(w843) -> ("Err Device"=w841:string)
        n333 = call "Time Delay3"("error in (no error)"=w832) -> ("error out"=w831:errorcluster)  [unwired: 10 in]
        n334 = case shown="\"No Err\", Default" w841 {
          tunnel: w840 -> [w862 w870]
          tunnel: w846 -> [_ w869]
          tunnel: [w863 w868] -> w842
          tunnel: w831 -> [w864 w867]
          frame "Zaber" {
            # "Zabe err do nothing, Msg?"
            n335 = Unbundle By Name(w862) -> ("Zaber Com"=w861:refnum<visa-resource-name>)
            n336 = One Button Dialog(message="Zaber Error") -> ()  [unwired: 1 in, 1 out]
            n337 = call <instrlib>:"Close.vi"("error in (no error)"=w864, "VISA resource name"=w861) -> ("error out"=w863:errorcluster)  [unwired: 9 in]
          }
          frame "No Err", Default {
            n338 = Unbundle By Name(w870) -> ("Zaber Com"=w866:refnum<visa-resource-name>)
            n339 = Unbundle By Name(w869) -> ()  [unwired: 1 out]
            n340 = Unbundle By Name(w869) -> ()  [unwired: 1 out]
            n341 = call <instrlib>:"Close.vi"("error in (no error)"=w867, "VISA resource name"=w866) -> ("error out"=w868:errorcluster)  [unwired: 9 in]
          }
        }
        n342 = Unbundle By Name(w840) -> ("MCU Com"=w834:refnum<visa-resource-name>, "LaserSysRef Out"=w838:refnum<k24>, "LaserControl Ref Out"=w839:refnum<k24>)
        n343 = case shown="\"No Err\", Default" w841 {
          tunnel: w842 -> [w859 w860]
          tunnel: [w858 w860] -> w837
          tunnel: w839 -> [w856 _]
          tunnel: w838 -> [w857 _]
          tunnel: w833 -> [w851 _]
          frame "No Err", Default {
            w852 = FALSE ("SysON")
            # "Laser Uninit here"
            n344 = call <vilib>:"Clear Errors.vi"("error in (no error)"=w859) -> ("error out"=w855:errorcluster)  [unwired: 5 in, 1 out]
            n345 = call "nLight-SystemON-ENA.vi"("ENA"=w852, "SysON"=w852, "Simulate (F)"=w851, "error in"=w855, "LaserControl Ref"=w856, "LaserSysRef"=w857) -> ("error out"=w854:errorcluster, "LaserSysRef Out"=w853:refnum<k24>)  [unwired: 3 in, 1 out]
            n346 = call "nLight-Disconnect.vi"("Simulate (F)"=w851, "error in"=w854, "LaserSysRef"=w853) -> ("error out"=w858:errorcluster)  [unwired: 8 in]
          }
          frame "Laser" {
            # "Laser Err, do nothing. There was a msg at \"Safe\" case"
          }
        }
        n347 = disable-structure shown="Enabled" {
          frame Disabled {
            n348 = One Button Dialog(message="Disable Laser, Home Axis, Uninit All") -> ()  [unwired: 1 in, 1 out]
          }
          frame Enabled {
          }
        }
        n349 = call "AR-Interlock-monitor-v2.vi"("Action"=AR-Interlock-monitor-comands."Close", "error in"=w837, "Inlk Com"=w834) -> ("error out"=w836:errorcluster)  [unwired: 4 in, 4 out]
        n350 = call "Stop-FGV.vi"("Action (RD)"=enum16{"Init", "WR", "RD"}."WR", "Action"=w847) -> ()  [unwired: 8 in, 2 out]
      }
    }
    "Instr Refs" <- w522
    n351 = local write "Axis params"(w518) -> ()
    n352 = Select(t="Quit" ("Action"), s=w529, f=w526) -> (s? t:f=w527:string)
    "Action" <- w524
  }
  n353 = while {
    tunnel: w1 -> [_]
    stop <- w876 stop-if-true
    n354 = call "AR-msg-vars-FGV.vi"("Action"=enum16{"Init", "WR", "RD"}."RD") -> ("error out"=w872:errorcluster, "msg-var"=w875:T1)  [unwired: 9 in]
    n355 = Wait (ms)(milliseconds to wait=u32 1) -> ()  [unwired: 1 out]
    n356 = local read "Accel Activ"() -> (w871:bool)
    n357 = Unbundle By Name(w875) -> ()  [unwired: 1 out]
    n358 = case shown="False" w871 {
      tunnel: w872 -> [_ w880]
      frame False {
      }
      frame True {
        n359 = call <vilib>:"Create File with Incrementing Suffix.vi"("error in (no error)"=w880, "file path"="Accel CSV File") -> ("error out"=w879:errorcluster, "actual path"=w878:path)  [unwired: 7 in, 1 out]
        n360 = call "py_accel.vi"("Time Target (s)"="Target Time (s)", "error in"=w879, "Accel CSV file"=w878, "COM"="Accel COM") -> ("File OK"=→"File OK":bool, "Com\nError"=→"Com\nError":bool)  [unwired: 6 in]
      }
    }
    n361 = call "Stop-FGV.vi"("Action (RD)"=enum16{"Init", "WR", "RD"}."RD") -> ("Out"=w876:bool)  [unwired: 9 in, 1 out]
  }
  n362 = call "Stop-FGV.vi"("Action (RD)"=enum16{"Init", "WR", "RD"}."WR", "error in"=w11, "Action"=TRUE) -> ("error out"=w8:errorcluster)  [unwired: 7 in, 1 out]
  n363 = call "Stop-FGV.vi"("Action (RD)"=enum16{"Init", "WR", "RD"}."WR", "error in"=w16, "Action"=TRUE) -> ("error out"=w9:errorcluster)  [unwired: 7 in, 1 out]
  n364 = Merge Errors(w10, w9, w8) -> (w4:errorcluster)
  n365 = call "AR-msg-vars-FGV.vi"("Action"=enum16{"Init", "WR", "RD"}."RD", "error in"=w4) -> ("error out"=→"error out":errorcluster, "msg-var"=→"msg-var at exit":T1)  [unwired: 8 in]
